vi "Esophogeal_HRME_Main_ImageCasting_VideoCapture.vi"() -> ()   [LabVIEW 2021]
uses:
  typeDefs/Esophogeal_Software_States.ctl
  <vilib>/Utility/miscctls.llb/LVAllMonitorsDisplayTypeDef.ctl
  <vilib>/DAQmx/read.llb/DAQmx Read (Digital 1D Bool NChan 1Samp 1Line).vi
  <extravilib>/ChannelInstances/High Speed Stream-str/_Read For Replicate.vi
  <extravilib>/ChannelInstances/High Speed Stream-a[.,.](u32)/_Read For Replicate.vi
  <extravilib>/ChannelInstances/High Speed Stream-a[.,.](u8)/_Read For Replicate.vi
  <extravilib>/ChannelInstances/Tag-bool/Read With Abort.vi
  <extravilib>/ChannelInstances/Tag-bool/Write With Abort.vi
  <vilib>/DAQmx/create/channels.llb/DAQmx Create Channel (DI-Digital Input).vi
  <vilib>/DAQmx/miscellaneous.llb/DAQmx Fill In Error Info.vi
  <extravilib>/ChannelInstances/Tag-bool/Instantiate.vi
  <extravilib>/ChannelInstances/High Speed Stream-str/Instantiate.vi
  <extravilib>/ChannelInstances/High Speed Stream-a[.,.](u32)/Instantiate.vi
  <extravilib>/ChannelInstances/High Speed Stream-str/)Channel.vi
  <extravilib>/ChannelInstances/High Speed Stream-str/Abort Signal/Init Signal.vi
  <extravilib>/ChannelInstances/High Speed Stream-a[.,.](u32)/)Channel.vi
  <extravilib>/ChannelInstances/High Speed Stream-a[.,.](u32)/Abort Signal/Init Signal.vi
  <extravilib>/ChannelInstances/High Speed Stream-a[.,.](u8)/Instantiate.vi
  <extravilib>/ChannelInstances/High Speed Stream-a[.,.](u8)/)Channel.vi
  <extravilib>/ChannelInstances/High Speed Stream-a[.,.](u8)/Abort Signal/Init Signal.vi
  <extravilib>/ChannelInstances/Tag-bool/EndpointRead.vi
  <extravilib>/ChannelInstances/Tag-bool/Endpoint.vi
  <vilib>/vision/driver/NI_Vision_Acquisition_Software.lvlib
  <resource>/objmgr/imaqdx.rc
  <extravilib>/ChannelInstances/High Speed Stream-a[.,.](u8).lvlib
  <extravilib>/ChannelInstances/High Speed Stream-str.lvlib
  <vilib>/vision/NI_Vision_Development_Module.lvlib
  <extravilib>/ChannelInstances/High Speed Stream-a[.,.](u32).lvlib
  <extravilib>/ChannelInstances/Tag-bool.lvlib
panel:
  out "Pause Status":bool
  in  "Tab Control":enum32{"Main Page", "Image Session Info"}(tab)
  in  "MTN Threshold:":enum16{"15.9", "24.0"}(ring)
  out "Endoscope Feed":T1(plugin-control)
  in  "Calibrate":bool
  out "Image Analysis Meter":dbl(slide) scale=0.0..100.0
  out "Saved Imaged Number":i32=1 caption="Number of Images Saved"
  out "Image Save Notification":string
  in  "Auto Gain":bool=TRUE
  in  "Auto Exposure":bool=TRUE
  in  "Save Button":bool
  out "Recording":bool
  in  "Play Button":bool
  in  "Pause Button":bool
  in  "Close Program":bool
  in  "HRME Gain":dbl(slide)=18.0 scale=0.0..30.0
  in  "HRME Exposure":dbl(slide)=7000.0 scale=100.0..80000.0
  out "HRME Image":T1(plugin-control)
  out "Software States":T2
  out "HRME Path":path
  out "HRME Scores":path
  out "Representative Images":path
  out "error out":errorcluster
  out "Patient Folder":path
  in  "Command File Location":path=path "C:/Users/EsophaHRME_Dell2/Documents/GitHub/Esophageal_HRME_Software/EsophagealDeployment/Multi_Task_Network/CommandFiles/LabVIEW/cmds.json"
  out "Display:All Monitors":T3
  out "Width":i16
  out "Height":i16=960
  out "WideField Path":path
  in  "Python Module Path":path=path "C:/Users/EsophaHRME_Dell2/Documents/GitHub/Esophageal_HRME_Software/EsophagealDeployment/Multi_Task_Network/mainv6.py"
  out "Log File Out":refnum<file>
  out "Timestamp":string
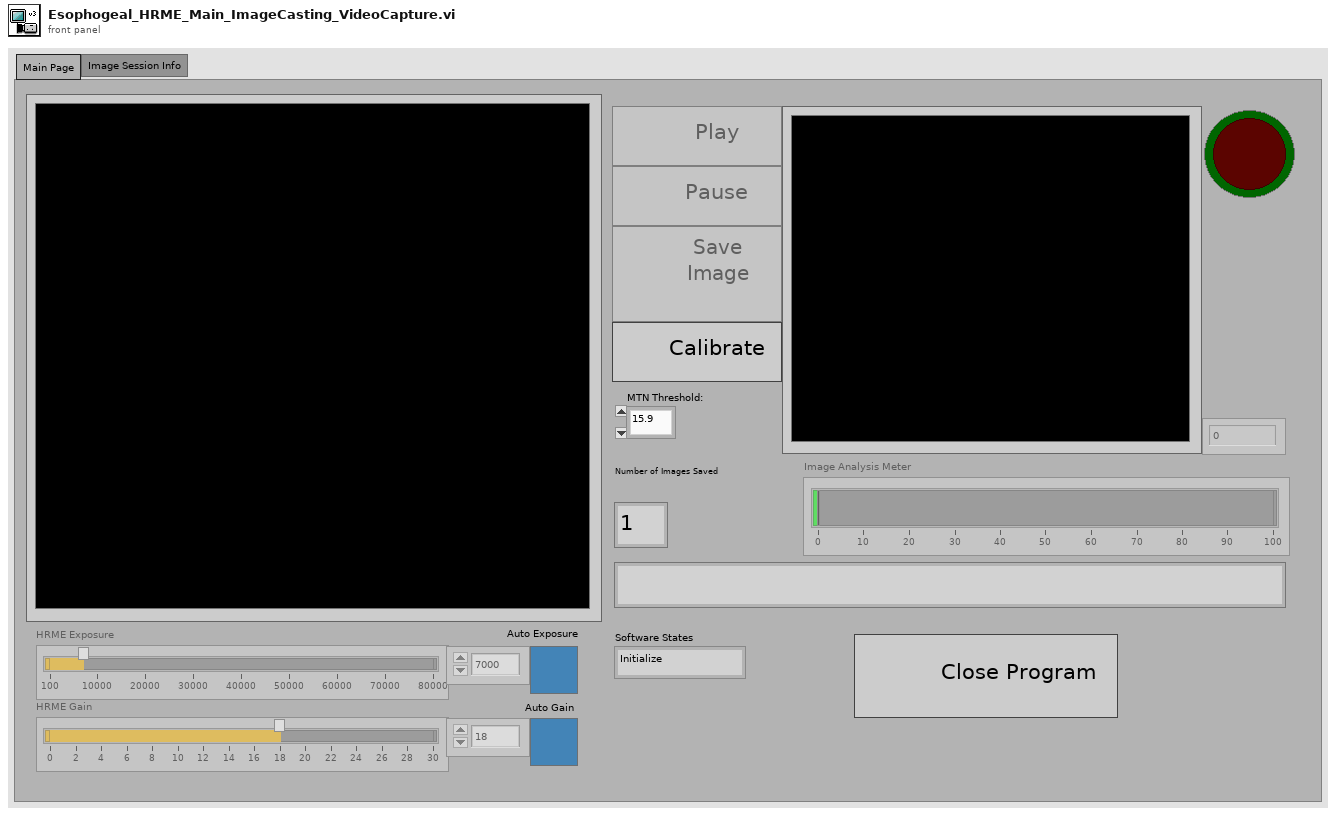
[diagram p1: front panel]
types:
  T1 = typedef "IMAQ Image.ctl" = refnum<image>
  T2 = typedef "Esophogeal_Software_States.ctl" = enum16{"Initialize", "Image Prep Screen", "Imaging", "Image Pause Screen", "Exit"}
  T3 = typedef "LVAllMonitorsDisplayTypeDef.ctl" = cluster{"Bounds":cluster{"Left":i16, "Top":i16, "Right":i16, "Bottom":i16}, "Depth":i16}[]
  T4 = enum8{"Enabled", "Disabled", "Disabled and Grayed Out"}
  T5 = enum16{"open", "replace", "create", "open or create", "replace or create", "replace or create with confirmation"}
  T6 = cluster{"Source":string, "Destination":string, "CMD":string, "Time":string}
  T7 = cluster{"Left":i32, "Top":i32, "Right":i32, "Bottom":i32}
  T8 = typedef "IMAQdx.ctl" = refnum<k21>
  T9 = cluster{"Bounds":cluster{"Left":i16, "Top":i16, "Right":i16, "Bottom":i16}, "Depth":i16}
  T10 = cluster{"Left":i16, "Top":i16, "Right":i16, "Bottom":i16}
  T11 = typedef "Image Type" = u32
  T12 = typedef "ROI Descriptor" = cluster{"Global Rectangle":i32[], "Contours":cluster{"ID":enum32{"External", "Internal"}, "Type":u32, "Coordinates":i32[]}[]}
  T13 = typedef "High Speed Stream-str.lvlib/)Channel.ctl" = refnum<queue>
  T14 = typedef "High Speed Stream-a[.,.](u8).lvlib/)Channel.ctl" = refnum<queue>
  T15 = typedef "Tag-bool.lvlib/))Channel.ctl" = refnum<queue>
  T16 = typedef "High Speed Stream-a[.,.](u32).lvlib/)Channel.ctl" = refnum<queue>
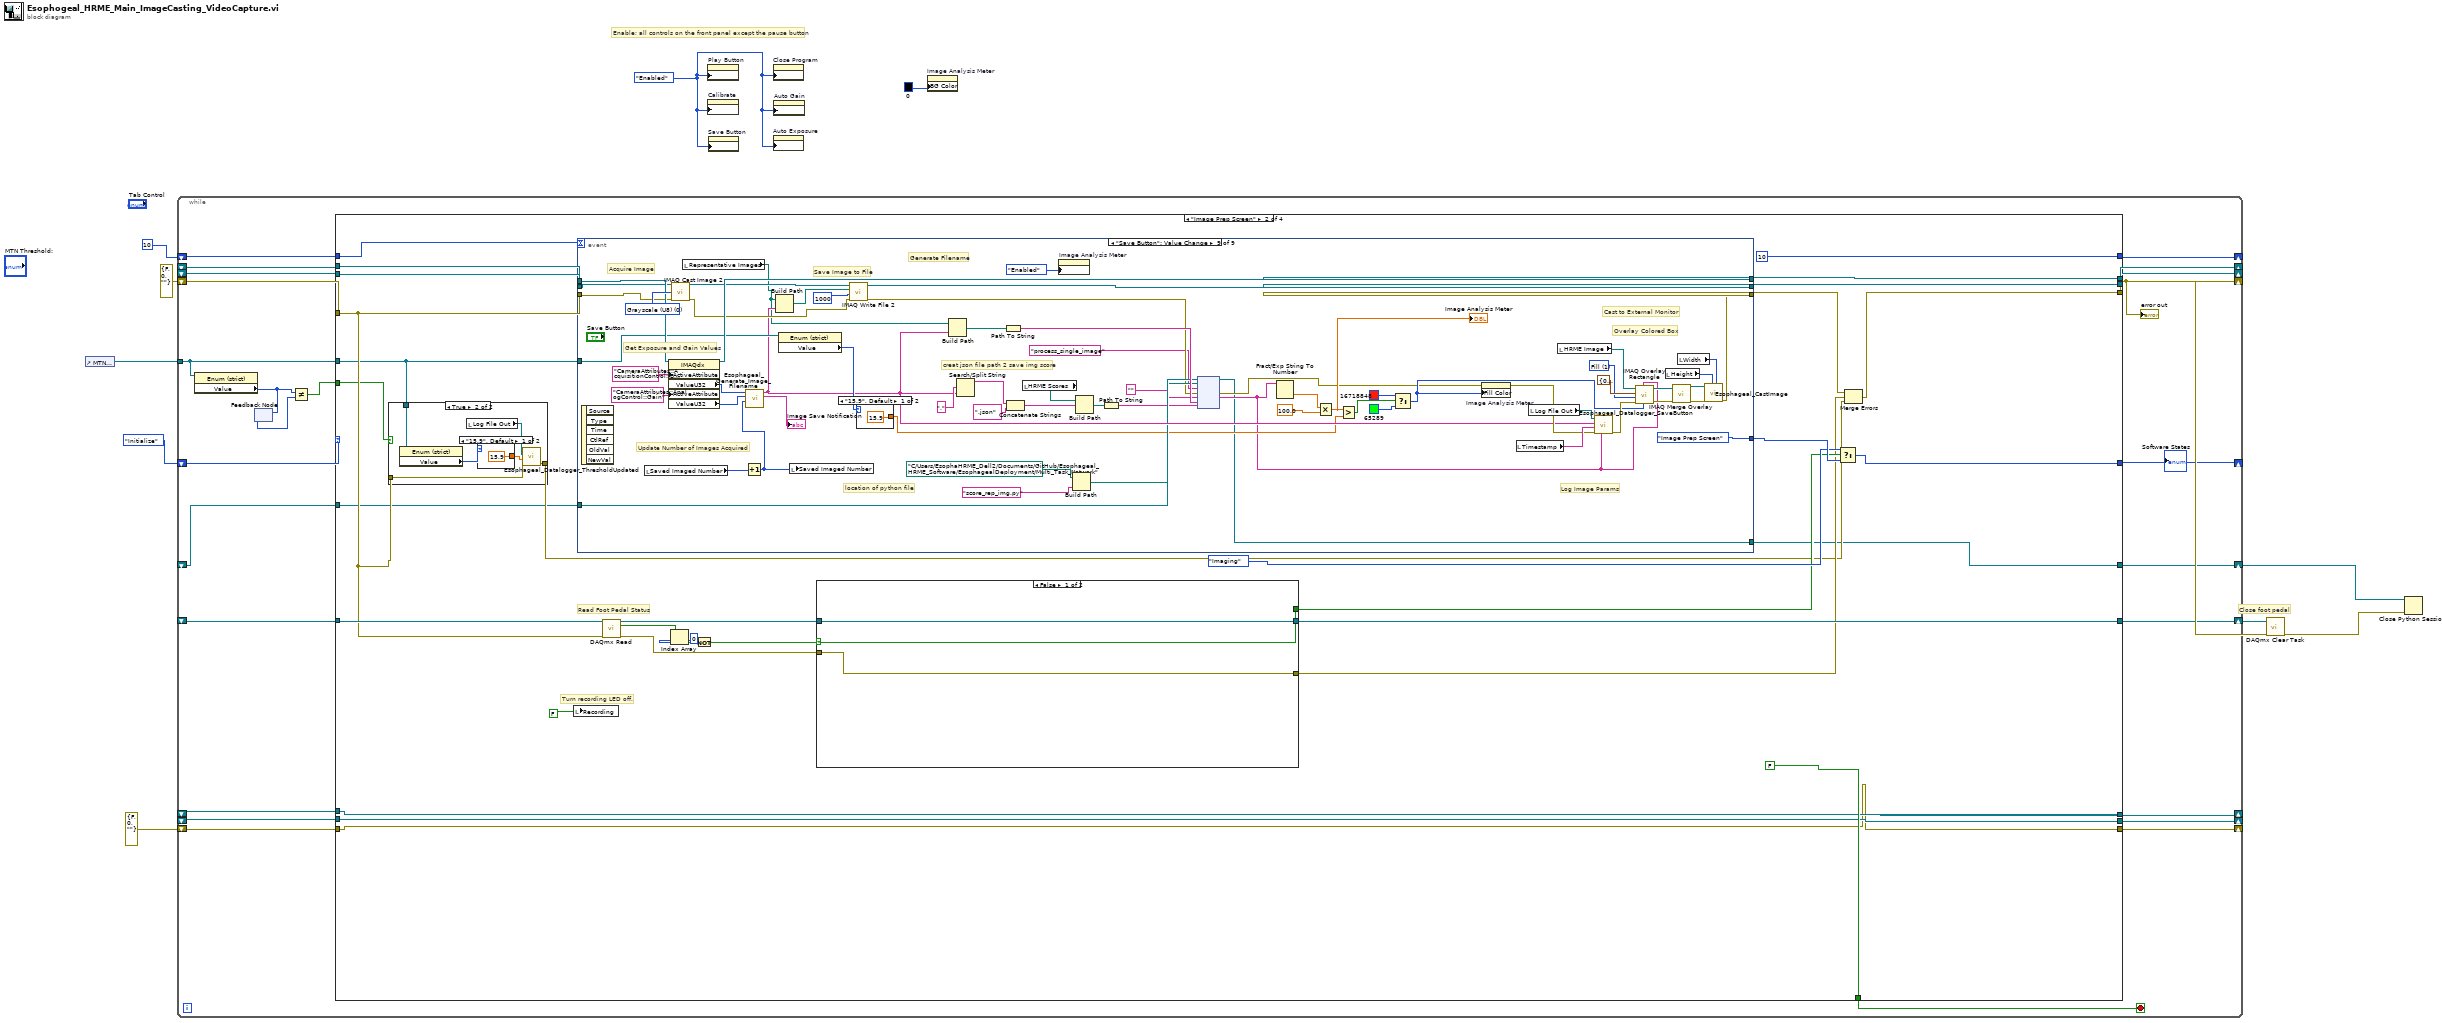
[diagram p0: block diagram]
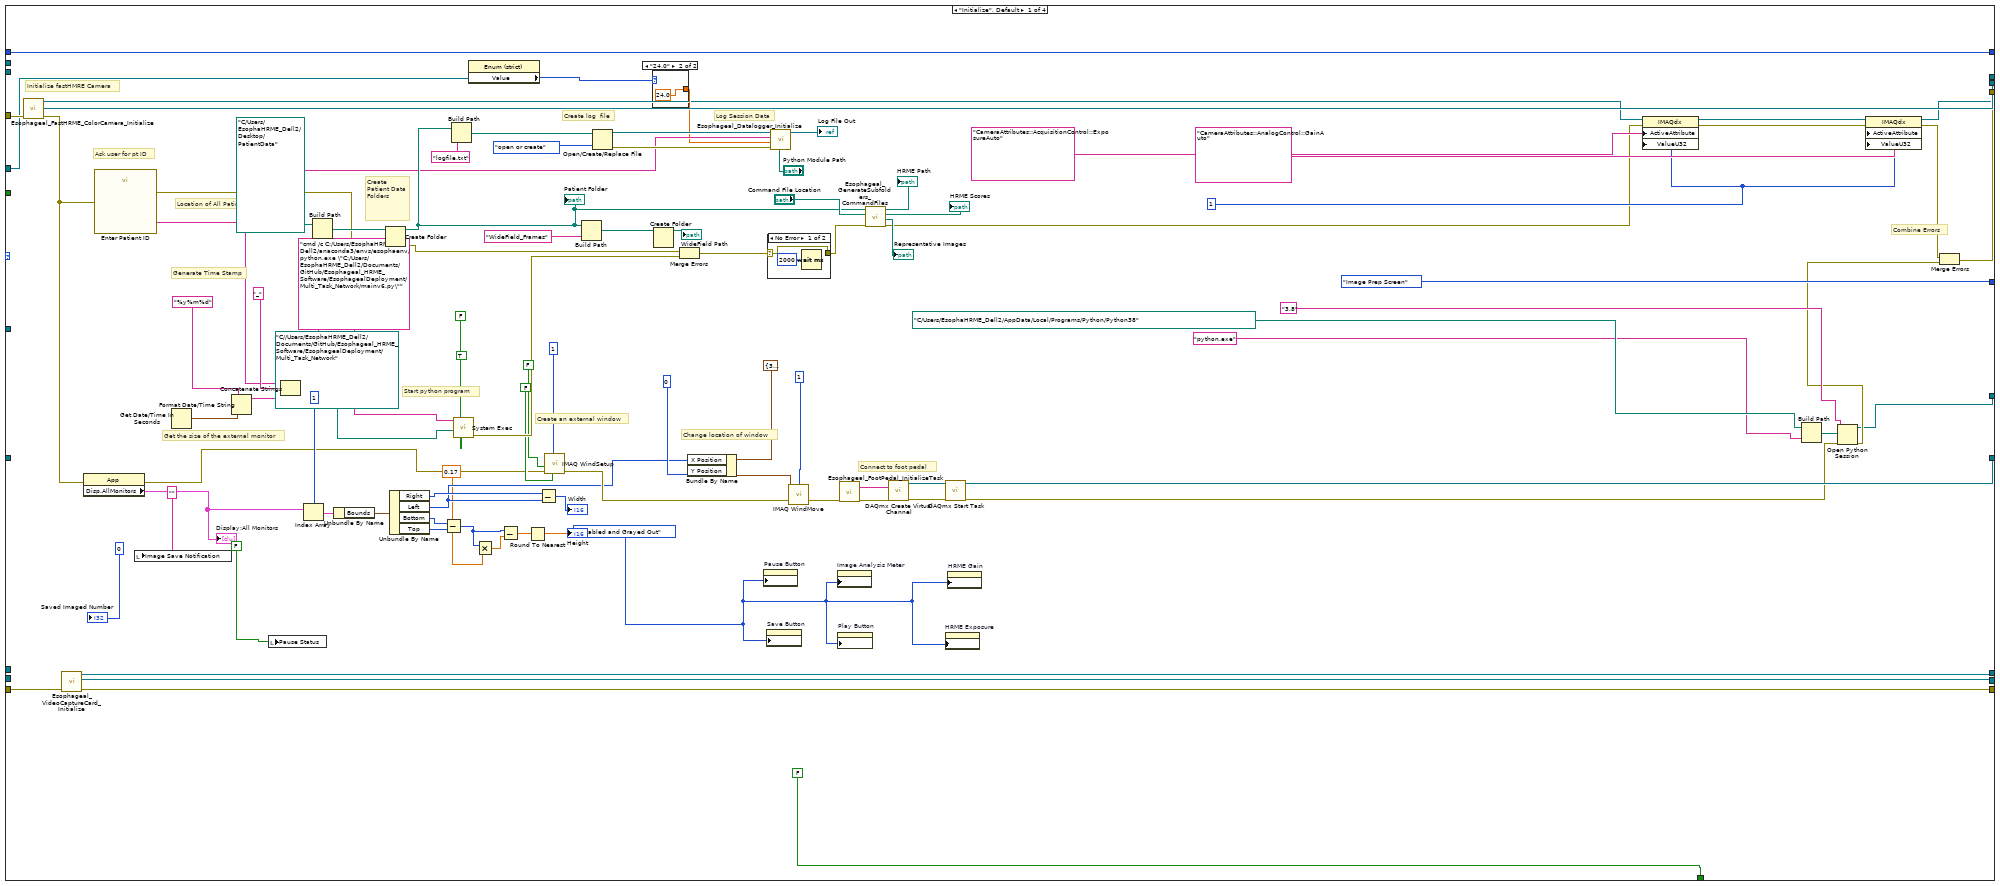
[diagram p2: hidden frame]
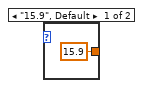
[diagram p3: hidden frame]
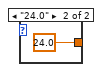
[diagram p6: hidden frame]
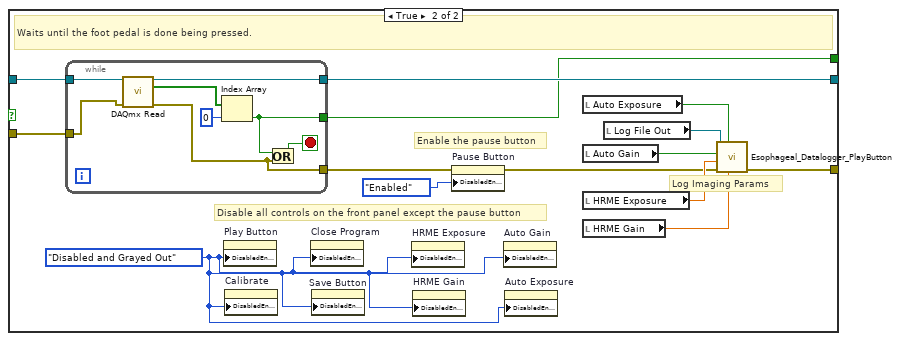
[diagram p7: hidden frame]
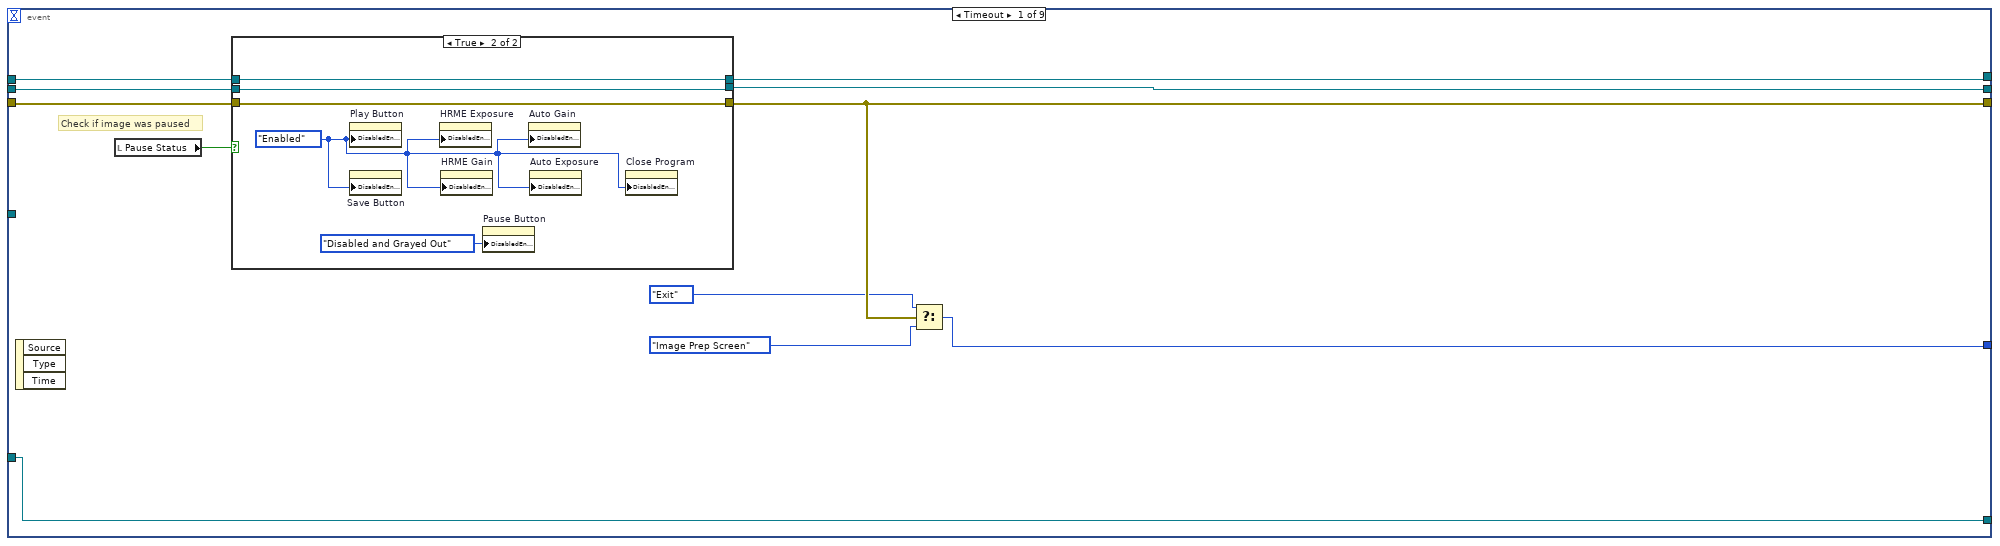
[diagram p8: hidden frame]
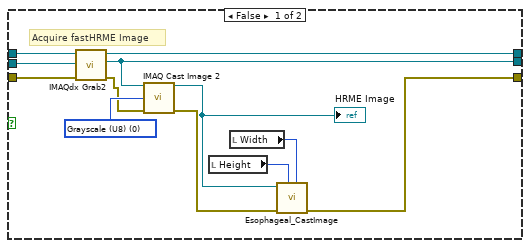
[diagram p9: hidden frame]
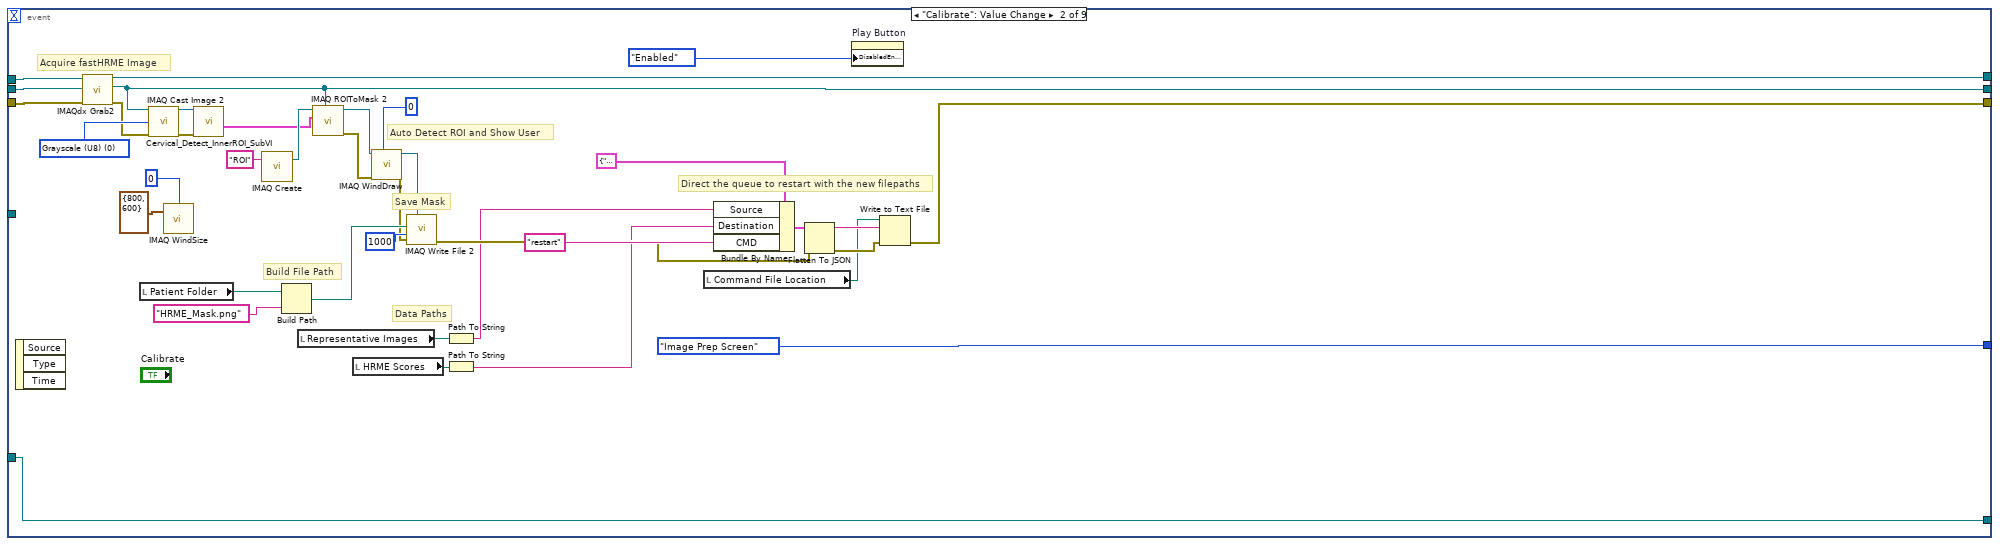
[diagram p10: hidden frame]
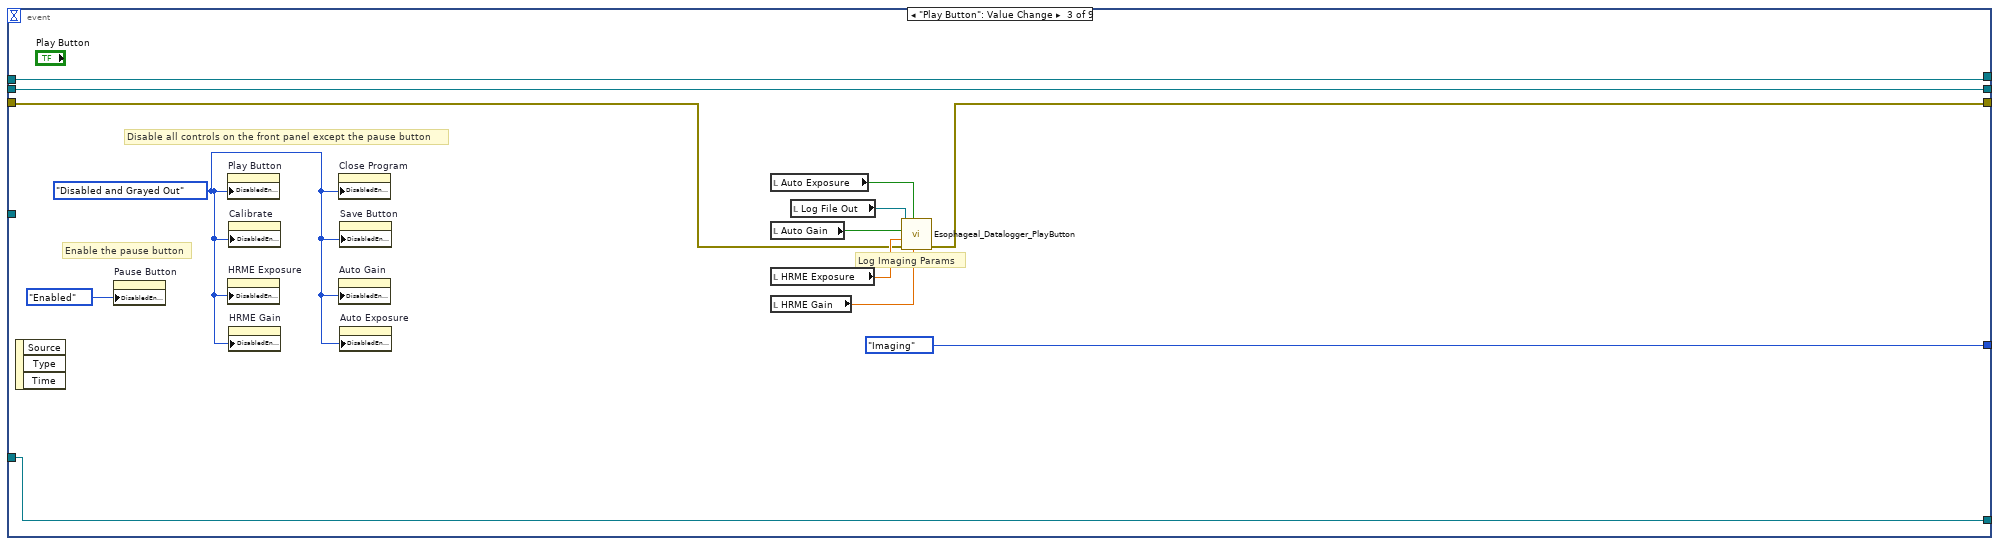
[diagram p11: hidden frame]
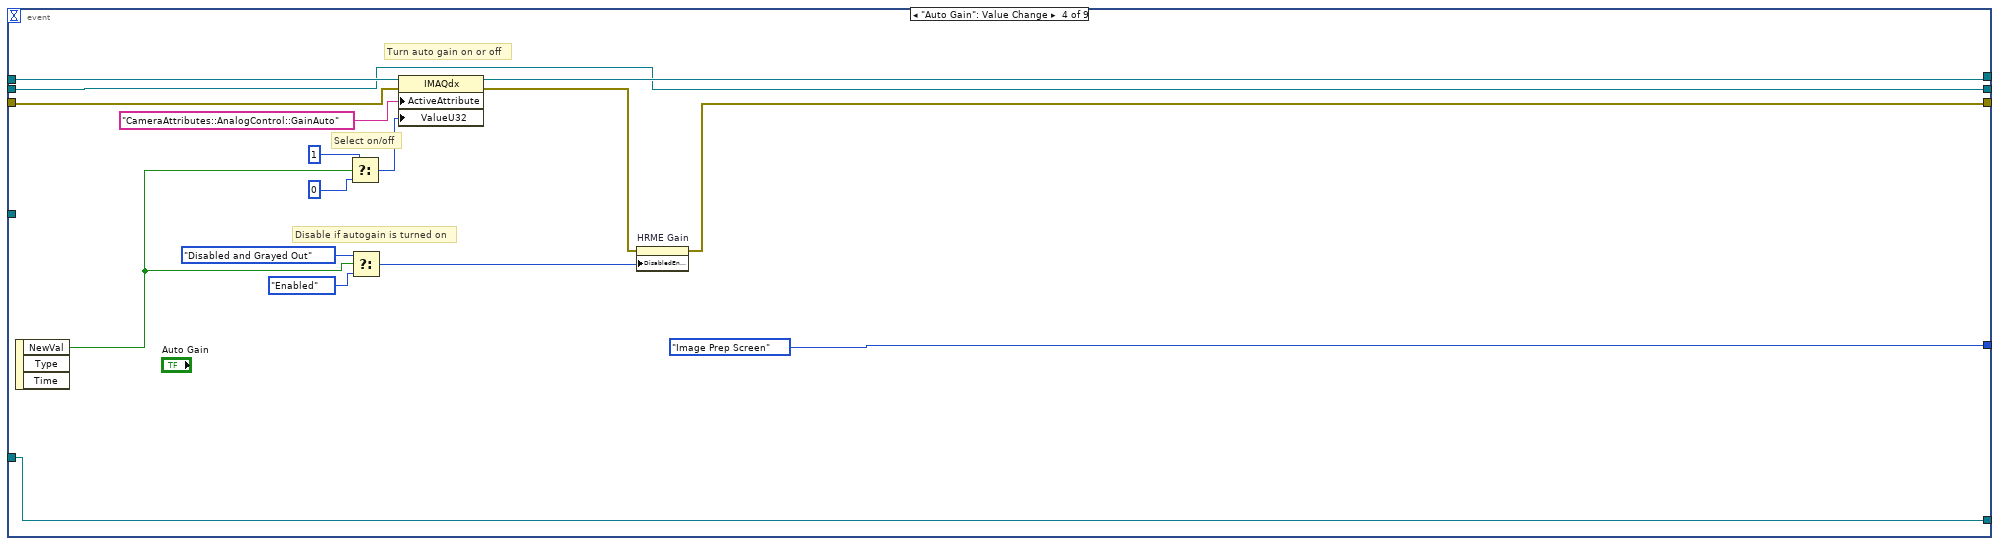
[diagram p12: hidden frame]
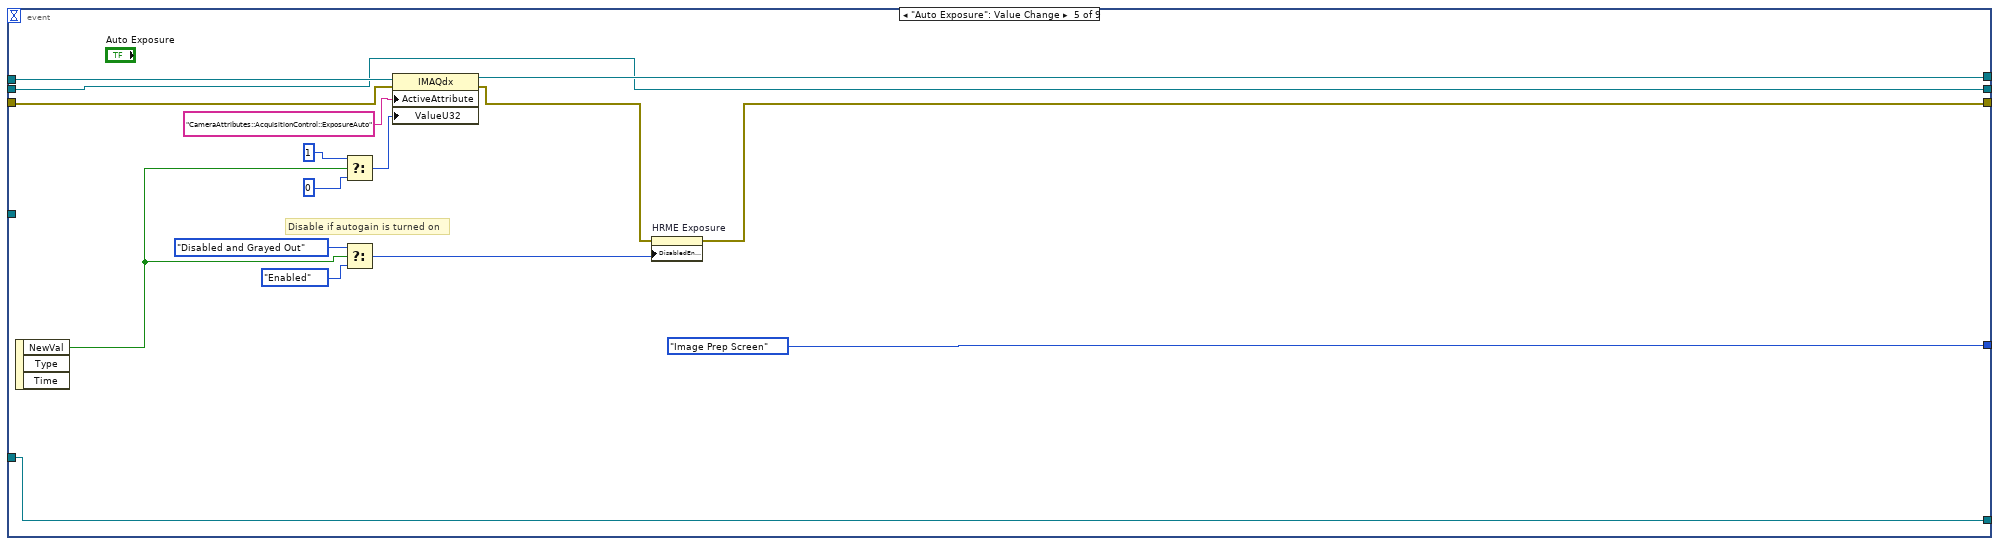
[diagram p13: hidden frame]
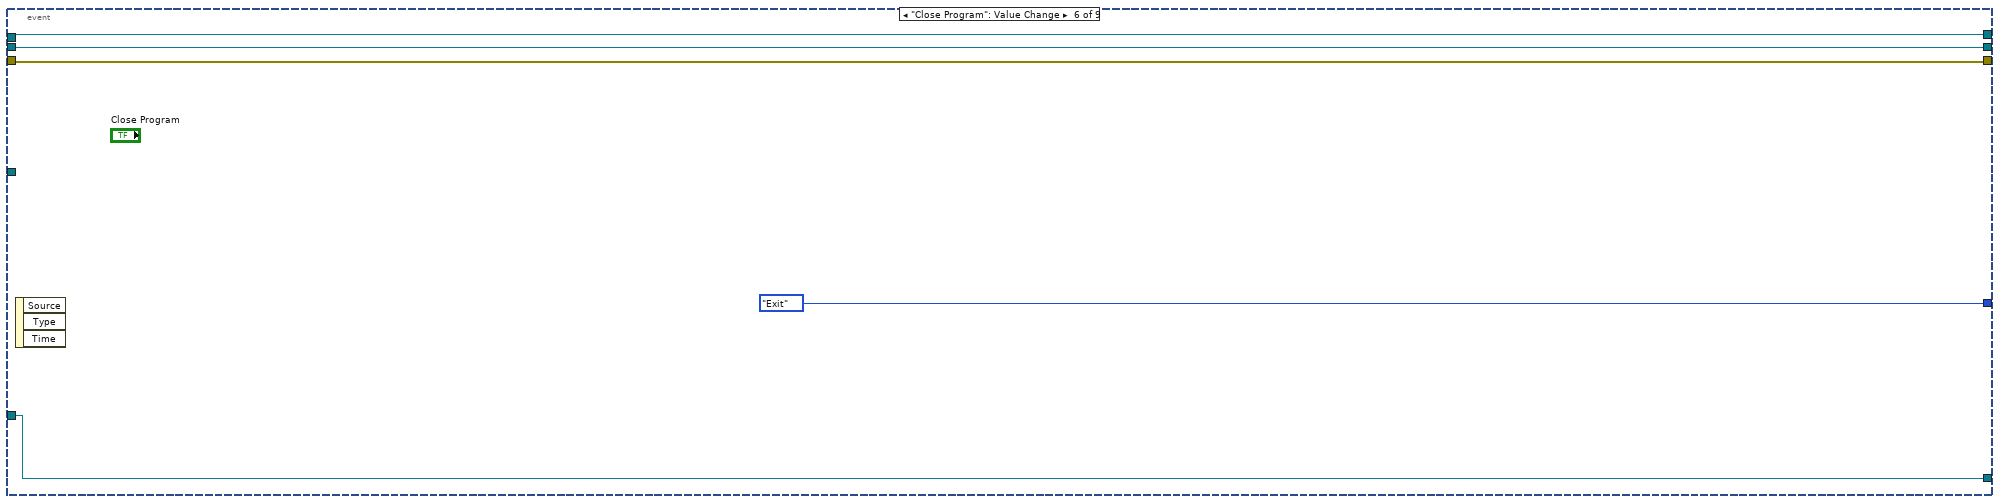
[diagram p14: hidden frame]
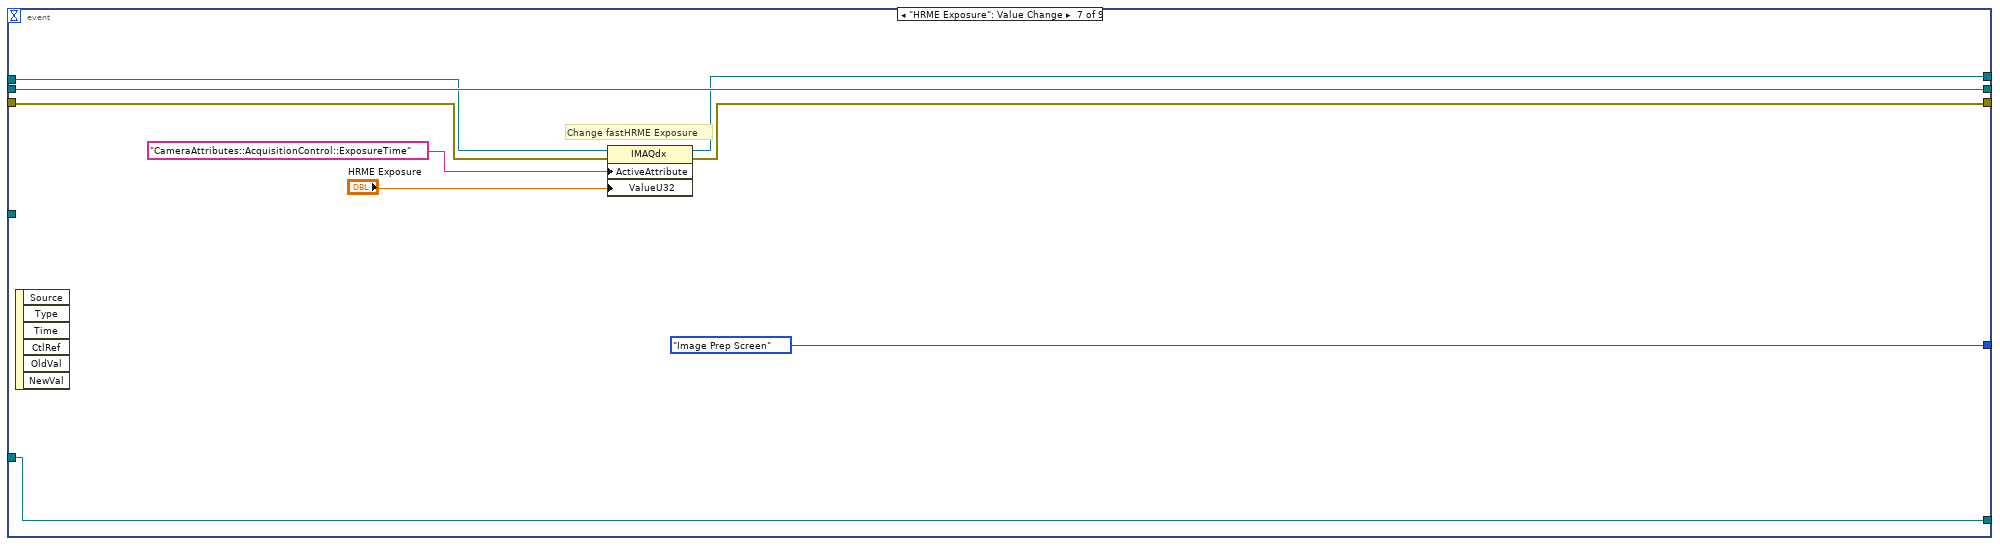
[diagram p15: hidden frame]
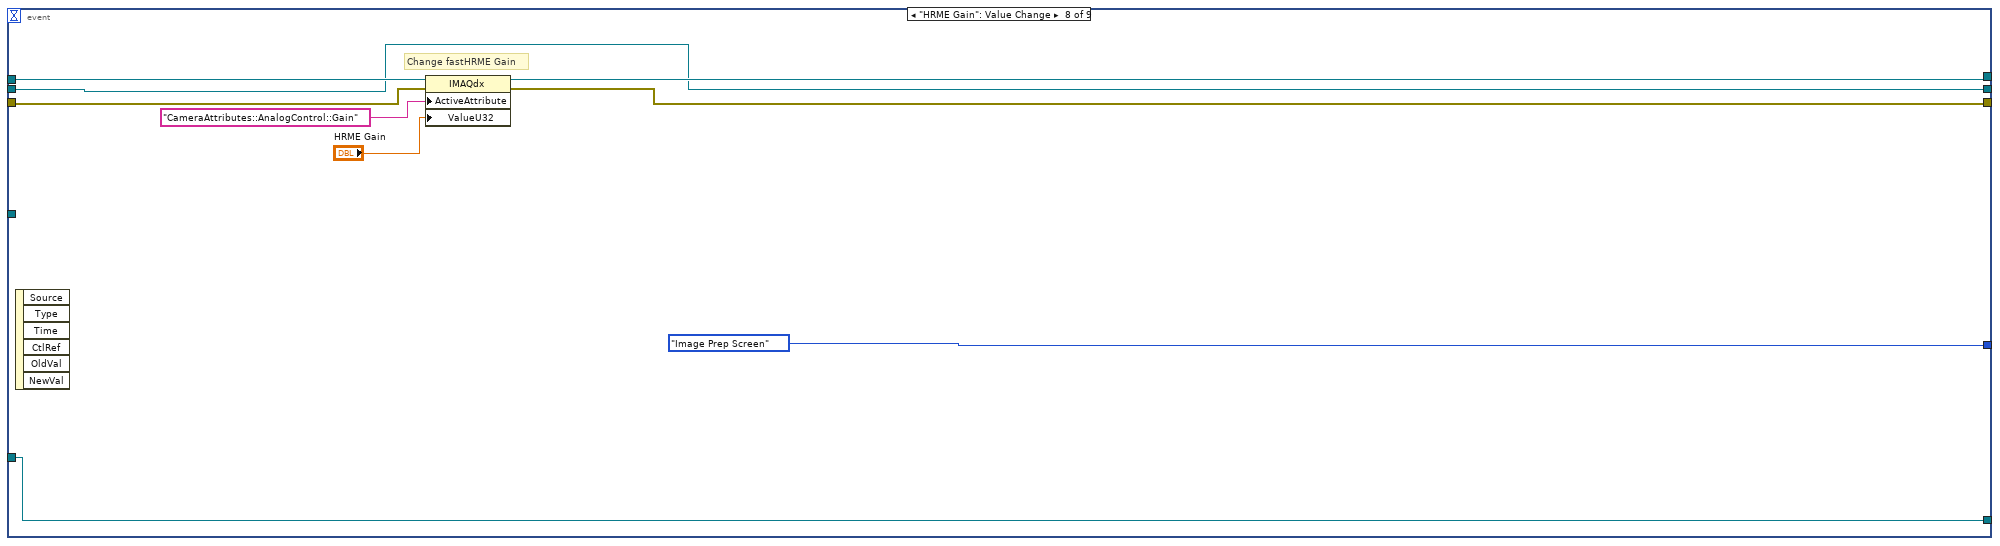
[diagram p16: hidden frame]
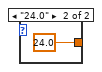
[diagram p17: hidden frame]
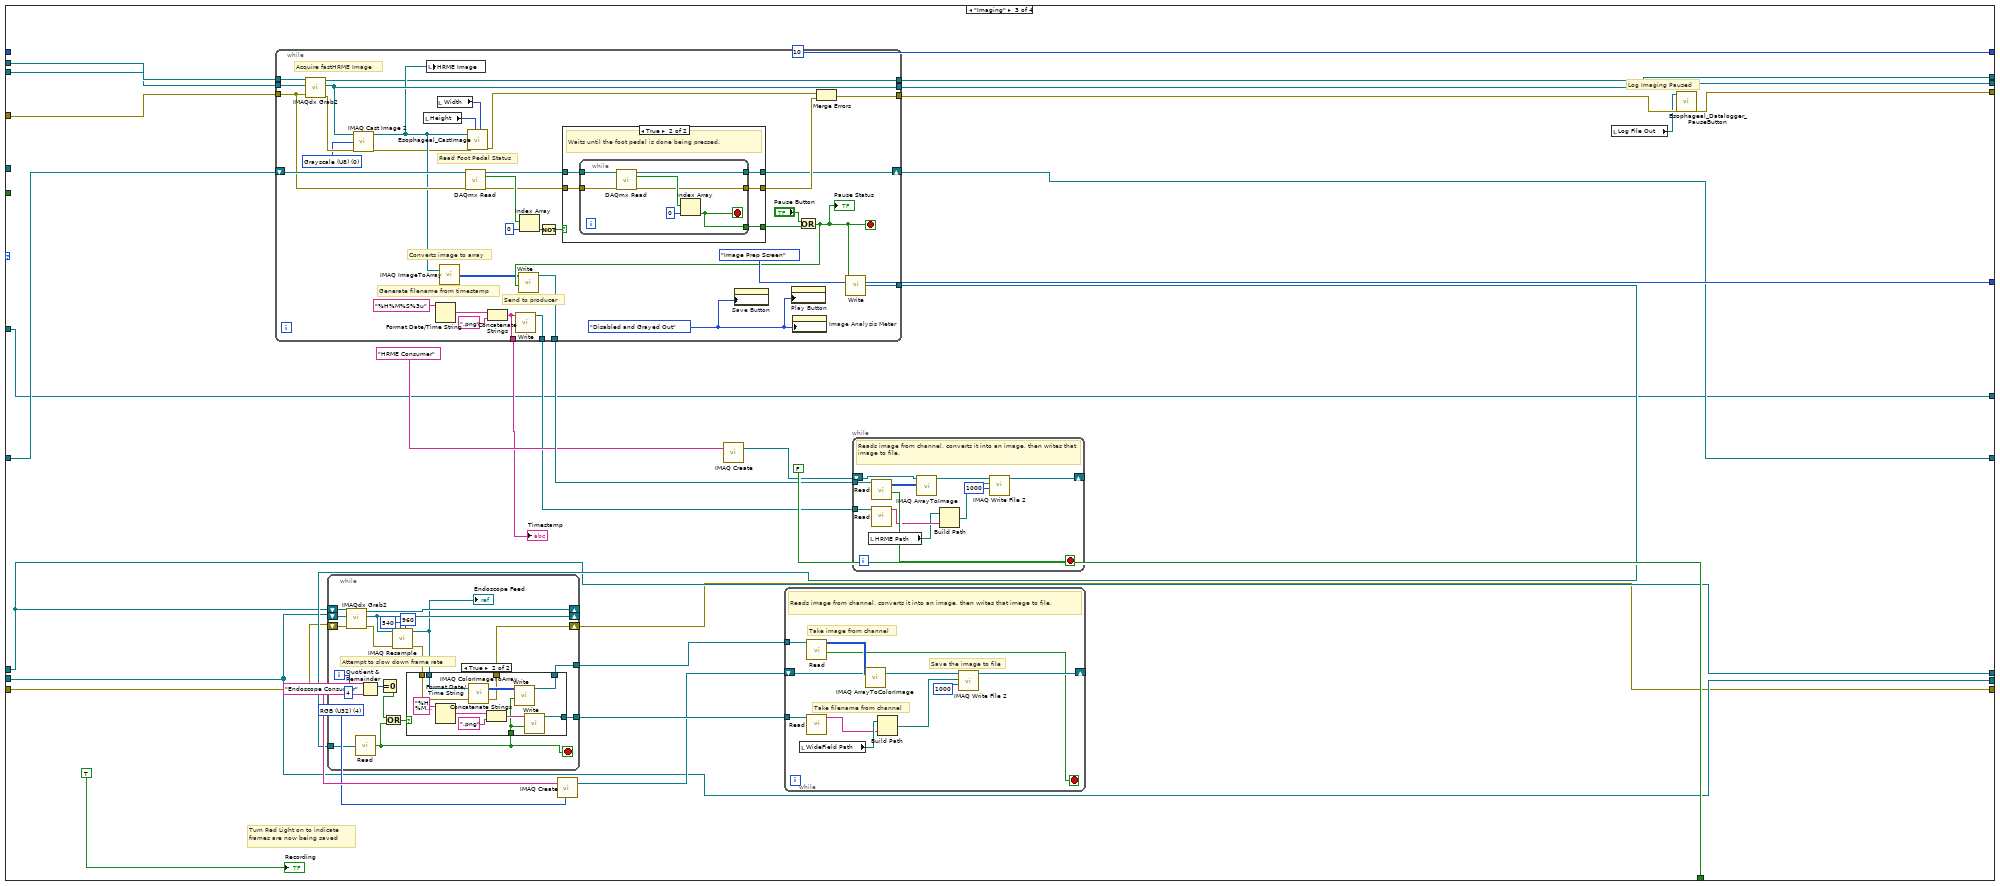
[diagram p18: hidden frame]
diagram:
  w3 = T4."Enabled" ("Disabled")
  # "Enable; all controls on the front panel except the pause button"
  # "Close foot pedal"
  n1 = control-ref of="MTN Threshold:"() -> (w4:refnum<vi>)
  n2 = while {
    shift-right: [w35] -> _
    shift-left: _ -> [w32]
    shift-right: [w34] -> _
    shift-left: _ -> [w31]
    shift-right: [w33] -> _
    shift-left: Esophogeal_Software_States."Initialize" ("Anal HRME States") -> [w36]
    shift-right: [w25] -> w9
    shift-left: errorcluster {"status"=FALSE, "code"=0, "source"=""} ("error IO") -> [w24]
    shift-right: [w28] -> w10
    shift-left: _ -> [w29]
    shift-right: [w26] -> _
    shift-left: 10 -> [w27]
    shift-right: [w21] -> _
    shift-left: _ -> [w22]
    shift-right: [w20] -> _
    shift-left: _ -> [w23]
    shift-right: [w18] -> _
    shift-left: errorcluster {"status"=FALSE, "code"=0, "source"=""} ("error in (no error)") -> [w19]
    tunnel: w4 -> [w17]
    shift-right: [w13] -> w2
    shift-left: _ -> [w12]
    stop <- w30 stop-if-true
    n3 = property class="Enum (strict)"(reference=w17) -> ("Value"=w16:enum16{"15.9", "24.0"})  [unwired: 1 in, 2 out]
    n4 = feedback-in #1(w16) -> ()
    n5 = feedback #1() -> (w15:enum16{"15.9", "24.0"})  [unwired: 1 in]
    n6 = Not Equal?(x=w16, y=w15) -> (x != y?=w14:bool)
    n7 = case shown="\"Image Prep Screen\"" w36 {
      tunnel: [w46 w166 w428 w554] -> w35
      tunnel: [w131 w165 w427 w553] -> w34
      tunnel: [Esophogeal_Software_States."Image Prep Screen" ("Anal HRME States") w162 Esophogeal_Software_States."Image Prep Screen" ("Anal HRME States") Esophogeal_Software_States."Exit" ("Anal HRME States")] -> w33
      tunnel: w24 -> [w129 w142 w412 w543]
      tunnel: w32 -> [_ w168 w430 w554]
      tunnel: w31 -> [_ w167 w429 w553]
      tunnel: [FALSE FALSE FALSE TRUE] -> w30
      tunnel: [w114 w146 w410 w541] -> w25
      tunnel: w29 -> [_ w158 w426 w551]
      tunnel: [w125 w153 w423 w551] -> w28
      tunnel: w27 -> [w124 w151 _ w550]
      tunnel: [w124 10 10 w550] -> w26
      tunnel: w19 -> [w65 w143 w407 w537]
      tunnel: w23 -> [_ w144 w405 w538]
      tunnel: w22 -> [_ w145 w406 w539]
      tunnel: [w62 w144 w405 w538] -> w20
      tunnel: [w63 w145 w406 w539] -> w21
      tunnel: [w64 w143 w404 w537] -> w18
      tunnel: w17 -> [w61 w139 _ _]
      tunnel: w14 -> [_ w140 _ _]
      tunnel: [w37 w137 w403 w536] -> w13
      tunnel: w12 -> [_ w138 w403 w536]
      frame "Initialize", Default {
        w50 = 1
        w44 = T4."Disabled and Grayed Out" ("Disabled")
        # "Log Session Data"
        # "Create log  file"
        # "Change location of window"
        # "Create an external window"
        # "Get the size of the external monitor"
        # "Start python program"
        # "Location of All Patient Data"
        # "Combine Errors"
        # "Create Patient Data Folders"
        # "Generate Time Stamp"
        # "Ask user for pt ID"
        # "Connect to foot pedal"
        # "Initialize fastHMRE Camera"
        n8 = call "Esophageal_FastHRME_ColorCamera_Initialize.vi"("error in (no error)"=w129) -> ("error out"=w91:errorcluster, "HRME Image Reference"=w131:T1, "OMS Camera Reference Out"=w47:T8)  [unwired: 8 in]
        n9 = call "Esophageal_VideoCaptureCard_Initialize.vi"("error in (no error)"=w65) -> ("error out"=w64:errorcluster, "Capture Card Image Out"=w62:T1, "Capture Card Camera Out"=w63:T8)  [unwired: 8 in]
        n10 = property class="App"(error in=w91) -> (error out=w80:errorcluster, "Disp.AllMonitors"=w98:T3)  [unwired: 1 in, 1 out]
        "Display:All Monitors" <- w98
        n11 = call "Enter Patient ID"("error in (no error)"=w91) -> ("Patient ID"=w66:string, "error out"=w115:errorcluster)  [unwired: 16 in, 1 out]
        n12 = local write "Image Save Notification"("" ("Image Save Notification")) -> ()
        n13 = Get Date/Time In Seconds() -> (seconds since 1Jan1904=w121:timestamp)
        n14 = Format Date/Time String(time format string (%c)="%y%m%d", seconds (now)=w121) -> (date/time string=w118:string)  [unwired: 1 in]
        n15 = local write "Pause Status"(FALSE ("Pause Status")) -> ()
        n16 = Concatenate Strings(w66, "_" ("string"), w118) -> (w117:string)
        n17 = Index Array(array=w98, index=1) -> (element=w96:T9)
        n18 = Build Path(base path=path "C:/Users/EsophaHRME_Dell2/Desktop/PatientData", name or relative path=w117) -> (appended path=w116:path)
        n19 = Unbundle By Name(w96) -> ("Bounds"=w95:T10)
        n20 = Create Folder(path (use dialog)=w116, error in=w115) -> (created path=w68:path, error out=w78:errorcluster)  [unwired: 1 in, 1 out]
        "Patient Folder" <- w68
        n21 = Unbundle By Name(w95) -> ("Right"=w94:i16, "Left"=w79:i16, "Bottom"=w93:i16, "Top"=w92:i16)
        n22 = Subtract(x=w93, y=w92) -> (x-y=w57:i16)
        n23 = Build Path(base path=w68, name or relative path="logfile.txt") -> (appended path=w74:path)
        n24 = call <vilib>:"System Exec.vi"("run minimized? (F)"=TRUE, "wait until completion? (T)"=FALSE, "working directory"=path "C://Users/EsophaHRME_Dell2/Documents/GitHub/Esophageal_HRME_Software/EsophagealDeployment/Multi_Task_Network", "command line"="cmd /c C:/Users/EsophaHRME_Dell2/anaconda3/envs/esophaenv/python.exe \"C:/Users/EsophaHRME_Dell2/Documents/GitHub/Esophageal_HRME_Software/EsophagealDeployment/Multi_Task_Network/mainv6.py\"") -> ("error out"=w103:errorcluster)  [unwired: 4 in, 3 out]
        n25 = property class="Enum (strict)"(reference=w61) -> ("Value"=w60:enum16{"15.9", "24.0"})  [unwired: 1 in, 2 out]
        n26 = Multiply(x=w57, y=0.17) -> (x*y=w56:dbl)
        n27 = Subtract(x=w57, y=w56) -> (x-y=w55:dbl)
        n28 = Round To Nearest(number=w55) -> (nearest integer value=→"Height":dbl)
        n29 = Subtract(x=w94, y=w79) -> (x-y=→"Width":i16)
        n30 = call "IMAQ WindSetup"("Window is floating? (No)"=FALSE, "Window Number (0...15)"=1, "error in (no error)"=w80, "Window has title bar? (Yes)"=FALSE) -> ("error out"=w81:errorcluster)  [unwired: 7 in]
        n31 = Build Path(base path=w68, name or relative path="WideField_Frames") -> (appended path=w76:path)
        n32 = Open/Create/Replace File(file path (use dialog)=w74, operation (0:open)=T5."open or create") -> (refnum out=w72:refnum<file>, error out=w71:errorcluster)  [unwired: 4 in, 1 out]
        n33 = case shown="\"24.0\"" w60 {
          tunnel: [15.9 24.0] -> w59
          frame "15.9", Default {
          }
          frame "24.0" {
          }
        }
        n34 = Create Folder(path (use dialog)=w76) -> (created path=→"WideField Path":path)  [unwired: 2 in, 2 out]
        n35 = Merge Errors(w78, w103) -> (w104:errorcluster)
        n36 = Bundle By Name(cluster=cluster{"X Position":i32, "Y Position":i32} {"X Position"=3840, "Y Position"=0} ("Coordinates (screen)"), "X Position"=w79, "Y Position"=0) -> (w86:cluster{"X Position":i32, "Y Position":i32})
        n37 = property on="Pause Button" class="Bool"("DisabledEnum"=w44) -> ()  [unwired: 2 in, 2 out]
        n38 = property on="Save Button" class="Bool"("DisabledEnum"=w44) -> ()  [unwired: 2 in, 2 out]
        n39 = case shown="No Error" w104 {
          selector: w104 -> [w134 w136]
          tunnel: [w134 w136] -> w108
          frame No Error {
            n40 = Wait (ms)(milliseconds to wait=u32 2000) -> ()  [unwired: 1 out]
          }
          frame Error {
          }
        }
        n41 = call "Esophageal_Datalogger_Initialize.vi"("Python Module Path"="Python Module Path", "error in (no error)"=w71, "MTN Threshold"=w59, "Patient ID"=w66, "Log File In"=w72) -> ("Log File Out"=→"Log File Out":refnum<file>)  [unwired: 5 in, 1 out]
        n42 = call "IMAQ WindMove"("Window Number (0...15)"=1, "Coordinates (screen)"=w86, "error in (no error)"=w81) -> ("error out"=w82:errorcluster)  [unwired: 2 in, 1 out]
        n43 = property on="Image Analysis Meter" class="Slide (strict)"("DisabledEnum"=w44) -> ()  [unwired: 2 in, 2 out]
        n44 = property on="Play Button" class="Bool"("DisabledEnum"=w44) -> ()  [unwired: 2 in, 2 out]
        n45 = call "Esophageal_FootPedal_InitializeTask.vi"("error in (no error)"=w82) -> ("error out"=w101:errorcluster, "Task Command"=w100:string)  [unwired: 9 in]
        n46 = call "Esophageal_GenerateSubfolders_CommandFiles.vi"("error in"=w108, "Command File Location"="Command File Location", "Patient Data Folder"=w68) -> ("error out"=w48:errorcluster, "Rep Image Path"=→"Representative Images":path, "HRME Scores"=→"HRME Scores":path, "HRME Path"=→"HRME Path":path)  [unwired: 5 in]
        n47 = call-poly <vilib>:"DAQmx Create Virtual Channel.vi"("lines"=w100, "error in"=w101) -> ("task out"=w126:refnum<k21>, "error out"=w127:errorcluster)  [unwired: 12 in]
        n48 = property on="HRME Exposure" class="Slide (strict)"("DisabledEnum"=w44) -> ()  [unwired: 2 in, 2 out]
        n49 = call <vilib>:"DAQmx Start Task.vi"("task/channels in"=w126, "error in"=w127) -> ("task out"=w125:refnum<k21>, "error out"=w39:errorcluster)  [unwired: 12 in]
        n50 = property on="HRME Gain" class="Slide (strict)"("DisabledEnum"=w44) -> ()  [unwired: 2 in, 2 out]
        n51 = property class="IMAQdx"(reference=w47, error in=w48, "ActiveAttribute"="CameraAttributes::AcquisitionControl::ExposureAuto", "ValueU32"=w50) -> (reference out=w49:T8, error out=w51:errorcluster)
        n52 = Build Path(base path=path "C:/Users/EsophaHRME_Dell2/AppData/Local/Programs/Python/Python38", name or relative path="python.exe") -> (appended path=w42:path)
        n53 = Open Python Session(python version="3.8", python path=w42, 3:w39) -> (session out=w37:refnum<k35>, error out=w38:errorcluster)
        n54 = property class="IMAQdx"(reference=w49, error in=w51, "ActiveAttribute"="CameraAttributes::AnalogControl::GainAuto", "ValueU32"=w50) -> (reference out=w46:T8, error out=w45:errorcluster)
        n55 = Merge Errors(w45, w38) -> (w114:errorcluster)
        "Saved Imaged Number" <- 0
      }
      frame "Image Prep Screen" {
        # "Turn recording LED off."
        # "Read Foot Pedal Status"
        n56 = case shown="True" w140 {
          tunnel: w142 -> [w169 w173]
          tunnel: [w169 w172] -> w141
          tunnel: w139 -> [_ w170]
          frame False {
          }
          frame True {
            n57 = property class="Enum (strict)"(reference=w170) -> ("Value"=w175:enum16{"15.9", "24.0"})  [unwired: 1 in, 2 out]
            n58 = local read "Log File Out"() -> (w171:refnum<file>)
            n59 = case shown="\"15.9\", Default" w175 {
              tunnel: [15.9 24.0] -> w174
              frame "15.9", Default {
              }
              frame "24.0" {
              }
            }
            n60 = call "Esophageal_Datalogger_ThresholdUpdated.vi"("error in"=w173, "MTN Threshold"=w174, "Log File In"=w171) -> ("error out"=w172:errorcluster)  [unwired: 7 in, 1 out]
          }
        }
        n61 = local write "Recording"(FALSE ("Recording")) -> ()
        n62 = event shown="[8] \"Save Button\": Value Change" {
          selector: _ -> [_ _ _ _ _ _ _ _ _]
          dyn-events: _ -> [_ _ _ _ _ _ _ _ _]
          timeout: w151 -> [_ _ _ _ _ _ _ _ _]
          tunnel: w168 -> [w213 w267 w280 w297 w310 w317 w325 w334 w385]
          tunnel: w167 -> [w211 w266 w279 w294 w307 w316 w326 w330 w384]
          tunnel: [w205 Esophogeal_Software_States."Image Prep Screen" ("Anal HRME States") Esophogeal_Software_States."Imaging" ("Anal HRME States") Esophogeal_Software_States."Image Prep Screen" ("Anal HRME States") Esophogeal_Software_States."Image Prep Screen" ("Anal HRME States") Esophogeal_Software_States."Exit" ("Anal HRME States") Esophogeal_Software_States."Image Prep Screen" ("Anal HRME States") Esophogeal_Software_States."Image Prep Screen" ("Anal HRME States") Esophogeal_Software_States."Image Prep Screen" ("Anal HRME States")] -> w161
          tunnel: [w212 w264 w280 w296 w309 w317 w324 w333 w395] -> w166
          tunnel: [w210 w242 w279 w294 w307 w316 w326 w330 w398] -> w165
          tunnel: w142 -> [w209 w265 w271 w295 w308 w315 w321 w331 w383]
          tunnel: [w206 w250 w270 w285 w303 w315 w320 w332 w380] -> w147
          tunnel: w139 -> [_ _ _ _ _ _ _ _ w367]
          tunnel: w138 -> [w203 w231 w269 w282 w298 w314 w319 w328 w353]
          tunnel: [w203 w231 w269 w282 w298 w314 w319 w328 w337] -> w137
          event Timeout {
            # "Check if image was paused"
            n63 = event-data() -> ()  [unwired: 1 in, 3 out]
            n64 = local read "Pause Status"() -> (w208:bool)
            n65 = case shown="True" w208 {
              tunnel: w213 -> [w225 w230]
              tunnel: [w224 w230] -> w212
              tunnel: w211 -> [w223 w229]
              tunnel: [w221 w229] -> w210
              tunnel: w209 -> [w222 w227]
              tunnel: [w216 w227] -> w206
              frame False {
                w220 = T11 0 items=["Grayscale (U8)", "Grayscale (I16)", "Grayscale (SGL)", "Complex (CSG)", "RGB (U32)", "HSL (U32)", "RGB (U64)", "Grayscale (U16)"] ("Image Type")
                # "Acquire fastHRME Image"
                n66 = call <vilib>:"IMAQdx Grab2.vi"("error in"=w222, "Image In"=w223, "Session In"=w225) -> ("error out"=w218:errorcluster, "Image Out"=w221:T1, "Session Out"=w224:T8)  [unwired: 5 in, 1 out]
                n67 = call "IMAQ Cast Image 2"("Image Src"=w221, "Image Type"=w220, "error in (no error)"=w218) -> ("Image Dst Out"=w219:T1, "error out"=w217:errorcluster)  [unwired: 11 in]
                "HRME Image" <- w219
                n68 = local read "Height"() -> (w215:i16)
                n69 = local read "Width"() -> (w214:i16)
                n70 = call "Esophageal_CastImage.vi"("X Resolution"=w214, "Y Resolution"=w215, "error in (no error)"=w217, "Image In"=w219) -> ("error out"=w216:errorcluster)  [unwired: 7 in]
              }
              frame True {
                w226 = T4."Enabled" ("Disabled")
                n71 = property on="Play Button" class="Bool"("DisabledEnum"=w226) -> ()  [unwired: 2 in, 2 out]
                n72 = property on="Save Button" class="Bool"("DisabledEnum"=w226) -> ()  [unwired: 2 in, 2 out]
                n73 = property on="HRME Exposure" class="Slide (strict)"("DisabledEnum"=w226) -> ()  [unwired: 2 in, 2 out]
                n74 = property on="HRME Gain" class="Slide (strict)"("DisabledEnum"=w226) -> ()  [unwired: 2 in, 2 out]
                n75 = property on="Pause Button" class="Bool"("DisabledEnum"=T4."Disabled and Grayed Out" ("Disabled")) -> ()  [unwired: 2 in, 2 out]
                n76 = property on="Auto Gain" class="Bool (strict)"("DisabledEnum"=w226) -> ()  [unwired: 2 in, 2 out]
                n77 = property on="Auto Exposure" class="Bool (strict)"("DisabledEnum"=w226) -> ()  [unwired: 2 in, 2 out]
                n78 = property on="Close Program" class="Bool"("DisabledEnum"=w226) -> ()  [unwired: 2 in, 2 out]
              }
            }
            n79 = Select(t=Esophogeal_Software_States."Exit" ("Anal HRME States"), s=w206, f=Esophogeal_Software_States."Image Prep Screen" ("Anal HRME States")) -> (s? t:f=w205:T2)
          }
          event "Calibrate": Value Change {
            w268 = T11 0 items=["Grayscale (U8)", "Grayscale (I16)", "Grayscale (SGL)", "Complex (CSG)", "RGB (U32)", "HSL (U32)", "RGB (U64)", "Grayscale (U16)"] ("Image Type")
            # "Auto Detect ROI and Show User"
            # "Data Paths"
            # "Direct the queue to restart with the new filepaths"
            # "Build File Path"
            # "Save Mask"
            # "Acquire fastHRME Image"
            n80 = event-data() -> ()  [unwired: 1 in, 3 out]
            n81 = call <vilib>:"IMAQdx Grab2.vi"("error in"=w265, "Image In"=w266, "Session In"=w267) -> ("error out"=w256:errorcluster, "Image Out"=w242:T1, "Session Out"=w264:T8)  [unwired: 5 in, 1 out]
            n82 = local read "Patient Folder"() -> (w262:path)
            n83 = call "IMAQ Cast Image 2"("Image Src"=w242, "Image Type"=w268, "error in (no error)"=w256) -> ("Image Dst Out"=w233:T1, "error out"=w234:errorcluster)  [unwired: 11 in]
            n84 = call "IMAQ WindSize"("Width & Height"=cluster{"Width":i32, "Height":i32} {"Width"=800, "Height"=600}, "Window Number"=0) -> ()  [unwired: 4 in, 3 out]
            n85 = call "Cervical_Detect_InnerROI_SubVI.vi"("error in"=w234, "Raw Image"=w233) -> ("ROI Descriptor"=w232:T12)  [unwired: 6 in, 3 out]
            n86 = call "IMAQ Create"("Image Name"="ROI") -> ("New Image"=w257:T1)  [unwired: 4 in, 1 out]
            n87 = Build Path(base path=w262, name or relative path="HRME_Mask.png") -> (appended path=w260:path)
            n88 = local read "Representative Images"() -> (w247:path)
            n89 = call "IMAQ ROIToMask 2"("Image Model"=w242, "ROI Descriptor"=w232, "Image"=w257) -> ("error out"=w237:errorcluster, "Image Out"=w238:T1)  [unwired: 6 in, 1 out]
            n90 = local read "HRME Scores"() -> (w246:path)
            n91 = call "IMAQ WindDraw"("Window Number (0...15)"=0, "error in (no error)"=w237, "Image"=w238) -> ("error out"=w235:errorcluster, "Image Out (duplicate)"=w236:T1)  [unwired: 7 in]
            n92 = call-poly "IMAQ Write File 2"("error in (no error)"=w235, "Image Quality"=u32 1000, "File Path"=w260, "Image"=w236) -> ("error out"=w252:errorcluster)  [unwired: 6 in, 1 out]
            n93 = Path To String(path=w247) -> (string=w245:string)
            n94 = Path To String(path=w246) -> (string=w244:string)
            n95 = local read "Command File Location"() -> (w248:path)
            n96 = Bundle By Name(cluster=T6 {"Source"="", "Destination"="", "CMD"="newfolders", "Time"="time"} ("Output JSON File"), "Source"=w245, "Destination"=w244, "CMD"="restart") -> (w254:T6)
            n97 = Flatten To JSON(anything=w254, error in (no error)=w252) -> (JSON string=w255:string, 11:w251:errorcluster)  [unwired: 1 in]
            n98 = property on="Play Button" class="Bool"("DisabledEnum"=T4."Enabled" ("Disabled")) -> ()  [unwired: 2 in, 2 out]
            n99 = Write to Text File(file (use dialog)=w248, text=w255, error in=w251) -> (error out=w250:errorcluster)  [unwired: 1 in, 2 out]
          }
          event "Play Button": Value Change {
            w277 = T4."Disabled and Grayed Out" ("Disabled")
            # "Log Imaging Params"
            # "Enable the pause button"
            # "Disable all controls on the front panel except the pause button"
            n100 = event-data() -> ()  [unwired: 1 in, 3 out]
            n101 = property on="Pause Button" class="Bool"("DisabledEnum"=T4."Enabled" ("Disabled")) -> ()  [unwired: 2 in, 2 out]
            n102 = property on="Play Button" class="Bool"("DisabledEnum"=w277) -> ()  [unwired: 2 in, 2 out]
            n103 = property on="HRME Exposure" class="Slide (strict)"("DisabledEnum"=w277) -> ()  [unwired: 2 in, 2 out]
            n104 = property on="Calibrate" class="Bool"("DisabledEnum"=w277) -> ()  [unwired: 2 in, 2 out]
            n105 = property on="HRME Gain" class="Slide (strict)"("DisabledEnum"=w277) -> ()  [unwired: 2 in, 2 out]
            n106 = property on="Close Program" class="Bool"("DisabledEnum"=w277) -> ()  [unwired: 2 in, 2 out]
            n107 = property on="Auto Gain" class="Bool (strict)"("DisabledEnum"=w277) -> ()  [unwired: 2 in, 2 out]
            n108 = property on="Save Button" class="Bool"("DisabledEnum"=w277) -> ()  [unwired: 2 in, 2 out]
            n109 = property on="Auto Exposure" class="Bool (strict)"("DisabledEnum"=w277) -> ()  [unwired: 2 in, 2 out]
            n110 = local read "Auto Exposure"() -> (w272:bool)
            n111 = local read "Auto Gain"() -> (w273:bool)
            n112 = local read "HRME Exposure"() -> (w274:dbl)
            n113 = local read "HRME Gain"() -> (w275:dbl)
            n114 = local read "Log File Out"() -> (w276:refnum<file>)
            n115 = call "Esophageal_Datalogger_PlayButton.vi"("Gain Value"=w275, "Auto Exposure Status"=w272, "error in (no error)"=w271, "Exposure Value"=w274, "Auto Gain Status"=w273, "Log File In"=w276) -> ("error out"=w270:errorcluster)  [unwired: 4 in, 1 out]
          }
          event "Auto Gain": Value Change {
            # "Disable if autogain is turned on"
            # "Select on/off"
            # "Turn auto gain on or off"
            n116 = event-data() -> ("NewVal"=w288:bool)  [unwired: 1 in, 2 out]
            n117 = Select(t=u32 1 ("ValueU32"), s=w288, f=u32 0 ("ValueU32")) -> (s? t:f=w291:u32)
            n118 = Select(t=T4."Disabled and Grayed Out" ("Disabled"), s=w288, f=T4."Enabled" ("Disabled")) -> (s? t:f=w287:T4)
            n119 = property class="IMAQdx"(reference=w297, error in=w295, "ActiveAttribute"="CameraAttributes::AnalogControl::GainAuto", "ValueU32"=w291) -> (reference out=w296:T8, error out=w286:errorcluster)
            n120 = property on="HRME Gain" class="Slide (strict)"(error in=w286, "DisabledEnum"=w287) -> (error out=w285:errorcluster)  [unwired: 1 in, 1 out]
          }
          event "Auto Exposure": Value Change {
            # "Disable if autogain is turned on"
            n121 = event-data() -> ("NewVal"=w301:bool)  [unwired: 1 in, 2 out]
            n122 = Select(t=u32 1 ("ValueU32"), s=w301, f=u32 0 ("ValueU32")) -> (s? t:f=w313:u32)
            n123 = Select(t=T4."Disabled and Grayed Out" ("Disabled"), s=w301, f=T4."Enabled" ("Disabled")) -> (s? t:f=w302:T4)
            n124 = property class="IMAQdx"(reference=w310, error in=w308, "ActiveAttribute"="CameraAttributes::AcquisitionControl::ExposureAuto", "ValueU32"=w313) -> (reference out=w309:T8, error out=w304:errorcluster)
            n125 = property on="HRME Exposure" class="Slide (strict)"(error in=w304, "DisabledEnum"=w302) -> (error out=w303:errorcluster)  [unwired: 1 in, 1 out]
          }
          event "Close Program": Value Change {
            n126 = event-data() -> ()  [unwired: 1 in, 3 out]
          }
          event "HRME Exposure": Value Change {
            # "Change fastHRME Exposure"
            n127 = event-data() -> ()  [unwired: 1 in, 6 out]
            n128 = property class="IMAQdx"(reference=w325, error in=w321, "ActiveAttribute"="CameraAttributes::AcquisitionControl::ExposureTime", "ValueU32"="HRME Exposure") -> (reference out=w324:T8, error out=w320:errorcluster)
          }
          event "HRME Gain": Value Change {
            # "Change fastHRME Gain"
            n129 = event-data() -> ()  [unwired: 1 in, 6 out]
            n130 = property class="IMAQdx"(reference=w334, error in=w331, "ActiveAttribute"="CameraAttributes::AnalogControl::Gain", "ValueU32"="HRME Gain") -> (reference out=w333:T8, error out=w332:errorcluster)
          }
          event "Save Button": Value Change {
            w373 = u32 1 items=["Frame", "Fill", "Highlight"] ("Drawing Mode (Frame)")
            w389 = T11 0 items=["Grayscale (U8)", "Grayscale (I16)", "Grayscale (SGL)", "Complex (CSG)", "RGB (U32)", "HSL (U32)", "RGB (U64)", "Grayscale (U16)"] ("Image Type")
            # "location of python file"
            # "creat json file path 2 save img score"
            # "Log Image Params"
            # "Overlay Colored Box"
            # "Cast to External Monitor"
            # "Update Number of Images Acquired"
            # "Generate Filename"
            # "Acquire Image"
            # "Get Exposure and Gain Values"
            # "Save Image to File"
            n131 = event-data() -> ()  [unwired: 1 in, 6 out]
            n132 = local read "Saved Imaged Number"() -> (w391:i32)
            n133 = property class="IMAQdx"(reference=w385, "ActiveAttribute"="CameraAttributes::AcquisitionControl::ExposureTime", "ActiveAttribute"="CameraAttributes::AnalogControl::Gain") -> (reference out=w395:T8, "ValueU32"=w394:u32, "ValueU32"=w393:u32)  [unwired: 1 in, 1 out]
            n134 = call "IMAQ Cast Image 2"("Image Src"=w384, "Image Type"=w389, "error in (no error)"=w383) -> ("Image Dst Out"=w388:T1, "error out"=w387:errorcluster)  [unwired: 11 in]
            n135 = local read "Representative Images"() -> (w358:path)
            n136 = Increment(x=w391) -> (x+1=w366:i32)
            n137 = call "Esophageal_Generate_Image_Filename.vi"("Image Number"=w366, "HRME Gain"=w393, "HRME Exposure"=w394) -> ("Notification Text"=→"Image Save Notification":string, "Image Filename"=w359:string)  [unwired: 7 in]
            n138 = Build Path(base path=w358, name or relative path=w359) -> (appended path=w400:path)
            n139 = property class="Enum (strict)"(reference=w367) -> ("Value"=w368:enum16{"15.9", "24.0"})  [unwired: 1 in, 2 out]
            n140 = local write "Saved Imaged Number"(w366) -> ()
            n141 = call-poly "IMAQ Write File 2"("error in (no error)"=w387, "Image Quality"=u32 1000, "File Path"=w400, "Image"=w388) -> ("error out"=w351:errorcluster, "Image Out (duplicate)"=w398:T1)  [unwired: 6 in]
            n142 = case shown="\"15.9\", Default" w368 {
              tunnel: [15.9 24.0] -> w343
              frame "15.9", Default {
              }
              frame "24.0" {
              }
            }
            n143 = Build Path(base path=w358, name or relative path=w359) -> (appended path=w360:path)
            n144 = Search/Split String(string=w359, search string/char (-)=".") -> (substring before match=w363:string)  [unwired: 1 in, 2 out]
            n145 = Path To String(path=w360) -> (string=w354:string)
            n146 = Concatenate Strings(w363, ".json") -> (w362:string)
            n147 = local read "HRME Scores"() -> (w357:path)
            n148 = property on="Image Analysis Meter" class="Slide (strict)"("DisabledEnum"=T4."Enabled" ("Disabled")) -> ()  [unwired: 2 in, 2 out]
            n149 = Build Path(base path=path "C:/Users/EsophaHRME_Dell2/Documents/GitHub/Esophageal_HRME_Software/EsophagealDeployment/Multi_Task_Network", name or relative path="score_rep_img.py") -> (appended path=w352:path)
            n150 = Build Path(base path=w357, name or relative path=w362) -> (appended path=w361:path)
            n151 = Path To String(path=w361) -> (string=w348:string)
            n152 = node(w353, w352, "process_single_image", w351, "", w354, w348) -> (w337:refnum<k35>, w338:errorcluster, w339:string)  [unwired: 2 in, 2 out]
            n153 = Fract/Exp String To Number(string=w339) -> (number=w344:dbl)  [unwired: 3 in, 1 out]
            n154 = Multiply(x=w344, y=100.0) -> (x*y=w341:dbl)
            "Image Analysis Meter" <- w341
            n155 = Greater?(x=w341, y=w343) -> (0:w347:bool)
            n156 = Select(t=u32 16718848, s=w347, f=u32 65289) -> (s? t:f=w340:u32)
            n157 = property on="Image Analysis Meter" class="Slide (strict)"(error in=w338, "Fill Color"=w340) -> (error out=w371:errorcluster)  [unwired: 1 in, 1 out]
            n158 = local read "Timestamp"() -> (w372:string)
            n159 = local read "Log File Out"() -> (w369:refnum<file>)
            n160 = local read "HRME Image"() -> (w379:T1)
            n161 = call "Esophageal_Datalogger_SaveButton.vi"("HRME Score"=w339, "error in (no error)"=w371, "Timestamp"=w372, "Image Name"=w359, "Log File In"=w369) -> ("error out"=w370:errorcluster)  [unwired: 5 in, 1 out]
            n162 = call "IMAQ Overlay Rectangle"("Color"=w340, "Group"=w339, "error in (no error)"=w370, "Drawing Mode (Frame)"=w373, "Rectangle"=T7 {"Left"=0, "Top"=0, "Right"=50, "Bottom"=50}, "Image"=w379) -> ("error out"=w375:errorcluster, "Image Out"=w378:T1)  [unwired: 4 in]
            n163 = local read "Height"() -> (w382:i16)
            n164 = call "IMAQ Merge Overlay"("error in (no error)"=w375, "Image Src"=w378) -> ("error out"=w376:errorcluster, "Image Dst Out"=w377:T1)  [unwired: 8 in]
            n165 = local read "Width"() -> (w381:i16)
            n166 = call "Esophageal_CastImage.vi"("X Resolution"=w381, "Y Resolution"=w382, "error in (no error)"=w376, "Image In"=w377) -> ("error out"=w380:errorcluster)  [unwired: 7 in]
          }
        }
        n167 = call-poly <vilib>:"DAQmx Read.vi"("task/channels in"=w158, "error in"=w142) -> ("task out"=w154:refnum<k21>, "data"=w157:bool[], "error out"=w149:errorcluster)  [unwired: 11 in]
        n168 = Index Array(array=w157, index=0) -> (element=w156:bool)
        n169 = Not(x=w156) -> (.not. x?=w155:bool)
        n170 = case shown="False" w155 {
          selector: w155 -> [w179 _]
          tunnel: w154 -> [w180 w194]
          tunnel: [w180 w193] -> w153
          tunnel: [w179 w192] -> w152
          tunnel: w149 -> [w178 w191]
          tunnel: [w178 w181] -> w148
          frame False {
          }
          frame True {
            w190 = T4."Disabled and Grayed Out" ("Disabled")
            # "Log Imaging Params"
            # "Enable the pause button"
            # "Disable all controls on the front panel except the pause button"
            # "Waits until the foot pedal is done being pressed."
            n171 = while {
              tunnel: w194 -> [w202]
              tunnel: [w201] -> w193
              tunnel: [w197] -> w192
              tunnel: w191 -> [w198]
              tunnel: [w195] -> w188
              stop <- w196 stop-if-true
              n172 = call-poly <vilib>:"DAQmx Read.vi"("task/channels in"=w202, "error in"=w198) -> ("task out"=w201:refnum<k21>, "data"=w199:bool[], "error out"=w195:errorcluster)  [unwired: 11 in]
              n173 = Index Array(array=w199, index=0) -> (element=w197:bool)
              n174 = Or(x=w197, y=w195) -> (x .or. y?=w196:bool)
            }
            n175 = property on="Play Button" class="Bool"("DisabledEnum"=w190) -> ()  [unwired: 2 in, 2 out]
            n176 = property on="Calibrate" class="Bool"("DisabledEnum"=w190) -> ()  [unwired: 2 in, 2 out]
            n177 = property on="Close Program" class="Bool"("DisabledEnum"=w190) -> ()  [unwired: 2 in, 2 out]
            n178 = property on="Save Button" class="Bool"("DisabledEnum"=w190) -> ()  [unwired: 2 in, 2 out]
            n179 = property on="HRME Exposure" class="Slide (strict)"("DisabledEnum"=w190) -> ()  [unwired: 2 in, 2 out]
            n180 = property on="HRME Gain" class="Slide (strict)"("DisabledEnum"=w190) -> ()  [unwired: 2 in, 2 out]
            n181 = property on="Pause Button" class="Bool"(error in=w188, "DisabledEnum"=T4."Enabled" ("Disabled")) -> (error out=w182:errorcluster)  [unwired: 1 in, 1 out]
            n182 = property on="Auto Gain" class="Bool (strict)"("DisabledEnum"=w190) -> ()  [unwired: 2 in, 2 out]
            n183 = property on="Auto Exposure" class="Bool (strict)"("DisabledEnum"=w190) -> ()  [unwired: 2 in, 2 out]
            n184 = local read "Auto Exposure"() -> (w183:bool)
            n185 = local read "Auto Gain"() -> (w184:bool)
            n186 = local read "HRME Exposure"() -> (w185:dbl)
            n187 = local read "HRME Gain"() -> (w186:dbl)
            n188 = local read "Log File Out"() -> (w187:refnum<file>)
            n189 = call "Esophageal_Datalogger_PlayButton.vi"("Gain Value"=w186, "Auto Exposure Status"=w183, "error in (no error)"=w182, "Exposure Value"=w185, "Auto Gain Status"=w184, "Log File In"=w187) -> ("error out"=w181:errorcluster)  [unwired: 4 in, 1 out]
          }
        }
        n190 = Select(t=Esophogeal_Software_States."Imaging" ("Anal HRME States"), s=w152, f=w161) -> (s? t:f=w162:T2)
        n191 = Merge Errors(w147, w148, w141) -> (w146:errorcluster)
      }
      frame "Imaging" {
        w413 = T11 4 items=["Grayscale (U8)", "Grayscale (I16)", "Grayscale (SGL)", "Complex (CSG)", "RGB (U32)", "HSL (U32)", "RGB (U64)", "Grayscale (U16)"] ("Image Type")
        # "Log Imaging Paused"
        # "Turn Red Light on to indicate frames are now being saved"
        n192 = while {
          tunnel: w430 -> [w520]
          tunnel: w429 -> [w519]
          tunnel: [w488] -> w428
          tunnel: [w498] -> w427
          tunnel: [w515] -> w411
          tunnel: w412 -> [w517]
          shift-right: [w512] -> w423
          shift-left: w426 -> [w518]
          tunnel: [w511] -> w422
          tunnel: [w509] -> w419
          tunnel: [w489] -> w414
          tunnel: [w487] -> w408
          stop <- w510 stop-if-true
          w495 = T4."Disabled and Grayed Out" ("Disabled")
          w496 = T11 0 items=["Grayscale (U8)", "Grayscale (I16)", "Grayscale (SGL)", "Complex (CSG)", "RGB (U32)", "HSL (U32)", "RGB (U64)", "Grayscale (U16)"] ("Image Type")
          # "Converts image to array"
          # "Generate filename from timestamp"
          # "Send to producer"
          # "Read Foot Pedal Status"
          # "Acquire fastHRME Image"
          n193 = call <vilib>:"IMAQdx Grab2.vi"("error in"=w517, "Image In"=w519, "Session In"=w520) -> ("error out"=w497:errorcluster, "Image Out"=w498:T1, "Session Out"=w488:T8)  [unwired: 5 in, 1 out]
          n194 = call "IMAQ Cast Image 2"("Image Src"=w498, "Image Type"=w496, "error in (no error)"=w497) -> ("Image Dst Out"=w492:T1, "error out"=w491:errorcluster)  [unwired: 11 in]
          n195 = local read "Height"() -> (w494:i16)
          n196 = local write "HRME Image"(w492) -> ()
          n197 = Format Date/Time String(time format string (%c)="%H%M%S%3u") -> (date/time string=w501:string)  [unwired: 2 in]
          n198 = local read "Width"() -> (w493:i16)
          n199 = call "IMAQ ImageToArray"("Image"=w492) -> ("Image Pixels (U8)"=w502:u8[][])  [unwired: 3 in, 4 out]
          n200 = call-poly <vilib>:"DAQmx Read.vi"("task/channels in"=w518, "error in"=w517) -> ("task out"=w504:refnum<k21>, "data"=w506:bool[], "error out"=w503:errorcluster)  [unwired: 11 in]
          n201 = call "Esophageal_CastImage.vi"("X Resolution"=w493, "Y Resolution"=w494, "error in (no error)"=w491, "Image In"=w492) -> ("error out"=w490:errorcluster)  [unwired: 7 in]
          n202 = Concatenate Strings(w501, ".png" ("string")) -> (w487:string)
          n203 = call <extravilib>:"Write.vi"("element"=w487) -> ("channel"=w509:T13)  [unwired: 8 in, 2 out]
          n204 = Index Array(array=w506, index=0) -> (element=w507:bool)
          n205 = Not(x=w507) -> (.not. x?=w505:bool)
          n206 = case shown="True" w505 {
            selector: w505 -> [w522 _]
            tunnel: w504 -> [w523 w528]
            tunnel: [w523 w527] -> w512
            tunnel: [w522 w524] -> w513
            tunnel: w503 -> [w521 w526]
            tunnel: [w521 w525] -> w516
            frame False {
            }
            frame True {
              # "Waits until the foot pedal is done being pressed."
              n207 = while {
                tunnel: w528 -> [w535]
                tunnel: [w534] -> w527
                tunnel: [w531] -> w524
                tunnel: w526 -> [w530]
                tunnel: [w529] -> w525
                stop <- w531 stop-if-true
                n208 = call-poly <vilib>:"DAQmx Read.vi"("task/channels in"=w535, "error in"=w530) -> ("task out"=w534:refnum<k21>, "data"=w532:bool[], "error out"=w529:errorcluster)  [unwired: 11 in]
                n209 = Index Array(array=w532, index=0) -> (element=w531:bool)
              }
            }
          }
          n210 = property on="Save Button" class="Bool"("DisabledEnum"=w495) -> ()  [unwired: 2 in, 2 out]
          n211 = property on="Play Button" class="Bool"("DisabledEnum"=w495) -> ()  [unwired: 2 in, 2 out]
          n212 = property on="Image Analysis Meter" class="Slide (strict)"("DisabledEnum"=w495) -> ()  [unwired: 2 in, 2 out]
          n213 = Or(x="Pause Button", y=w513) -> (x .or. y?=w510:bool)
          "Pause Status" <- w510
          n214 = call <extravilib>:"Write.vi"("last element? (F)"=w510, "element"=w502) -> ("channel"=w511:T14)  [unwired: 7 in, 2 out]
          n215 = Merge Errors(w490, w516) -> (w515:errorcluster)
          n216 = call <extravilib>:"Write.vi"("element"=w510) -> ("channel"=w489:T15)  [unwired: 1 out]
        }
        "Timestamp" <- w408
        n217 = while {
          shift-right: [w463] -> _
          shift-left: w406 -> [w462]
          shift-right: [w456] -> _
          shift-left: w405 -> [w461]
          shift-right: [w453] -> w404
          shift-left: w407 -> [w460]
          tunnel: [w459] -> w417
          tunnel: [w458] -> w416
          tunnel: w414 -> [w457]
          i -> [w449]
          stop <- w446 stop-if-true
          # "Attempt to slow down frame rate"
          n218 = call <vilib>:"IMAQdx Grab2.vi"("error in"=w460, "Image In"=w461, "Session In"=w462) -> ("error out"=w455:errorcluster, "Image Out"=w456:T1, "Session Out"=w463:T8)  [unwired: 5 in, 1 out]
          n219 = call <extravilib>:"Read.vi"("channel"=w457) -> ("element"=w446:bool)  [unwired: 1 in, 1 out]
          n220 = Quotient & Remainder(x=w449, y=4) -> (x-y*floor(x/y)=w447:i32)  [unwired: 1 out]
          n221 = Equal To 0?(x=w447) -> (x = 0?=w445:bool)
          n222 = Or(x=w445, y=w446) -> (x .or. y?=w444:bool)
          n223 = call "IMAQ Resample"("X Resolution"=960, "Y Resolution"=540, "error in (no error)"=w455, "Image Src"=w456) -> ("error out"=w454:errorcluster, "Image Dst Out"=w452:T1)  [unwired: 6 in]
          "Endoscope Feed" <- w452
          n224 = case shown="True" w444 {
            tunnel: [_ w474] -> w459
            tunnel: [_ w469] -> w458
            tunnel: w446 -> [_ w465]
            tunnel: w454 -> [w464 w468]
            tunnel: [w464 w467] -> w453
            tunnel: w452 -> [_ w466]
            frame False {
            }
            frame True {
              n225 = Format Date/Time String(time format string (%c)="%H%M%S%3u") -> (date/time string=w471:string)  [unwired: 2 in]
              n226 = call "IMAQ ColorImageToArray"("Image"=w466, "error in (no error)"=w468) -> ("Image Pixels (U32)"=w475:u32[][], "error out"=w467:errorcluster)  [unwired: 2 in, 1 out]
              n227 = Concatenate Strings(w471, ".png" ("string")) -> (w470:string)
              n228 = call <extravilib>:"Write.vi"("last element? (F)"=w465, "element"=w475) -> ("channel"=w474:T16)  [unwired: 7 in, 2 out]
              n229 = call <extravilib>:"Write.vi"("last element? (F)"=w465, "element"=w470) -> ("channel"=w469:T13)  [unwired: 7 in, 2 out]
            }
          }
        }
        n230 = call "IMAQ Create"("Image Name"="Endoscope Consumer", "Image Type"=w413) -> ("New Image"=w415:T1)  [unwired: 3 in, 1 out]
        n231 = call "IMAQ Create"("Image Name"="HRME Consumer") -> ("New Image"=w420:T1)  [unwired: 4 in, 1 out]
        n232 = while {
          tunnel: w417 -> [w443]
          tunnel: w416 -> [w442]
          shift-right: [w435] -> _
          shift-left: w415 -> [w440]
          stop <- w433 stop-if-true
          # "Take filename from channel"
          # "Take image from channel"
          # "Save the image to file"
          # "Reads image from channel, converts it into an image, then writes that image to file."
          n233 = local read "WideField Path"() -> (w439:path)
          n234 = call <extravilib>:"Read.vi"("channel"=w443) -> ("done?"=w433:bool, "element"=w441:u32[][])  [unwired: 6 in, 3 out]
          n235 = call <extravilib>:"Read.vi"("channel"=w442) -> ("element"=w438:string)  [unwired: 6 in, 4 out]
          n236 = call "IMAQ ArrayToColorImage"("Image Pixels (U32)"=w441, "Image"=w440) -> ("Image Out"=w436:T1)  [unwired: 3 in, 1 out]
          n237 = Build Path(base path=w439, name or relative path=w438) -> (appended path=w434:path)
          n238 = call-poly "IMAQ Write File 2"("Image Quality"=u32 1000, "File Path"=w434, "Image"=w436) -> ("Image Out (duplicate)"=w435:T1)  [unwired: 7 in, 1 out]
        }
        n239 = while {
          tunnel: w422 -> [w486]
          shift-right: [w482] -> _
          shift-left: w420 -> [w478]
          tunnel: w419 -> [w481]
          stop <- w485 stop-if-true
          # "Reads image from channel, converts it into an image, then writes that image to file."
          n240 = local read "HRME Path"() -> (w477:path)
          n241 = call <extravilib>:"Read.vi"("channel"=w486) -> ("done?"=w485:bool, "element"=w484:u8[][])  [unwired: 6 in, 3 out]
          n242 = call <extravilib>:"Read.vi"("channel"=w481) -> ("element"=w479:string)  [unwired: 6 in, 4 out]
          n243 = call "IMAQ ArrayToImage"("Image Pixels (U8)"=w484, "Image"=w478) -> ("Image Out"=w483:T1)  [unwired: 8 in, 1 out]
          n244 = Build Path(base path=w477, name or relative path=w479) -> (appended path=w480:path)
          n245 = call-poly "IMAQ Write File 2"("Image Quality"=u32 1000, "File Path"=w480, "Image"=w483) -> ("Image Out (duplicate)"=w482:T1)  [unwired: 7 in, 1 out]
        }
        n246 = local read "Log File Out"() -> (w409:refnum<file>)
        n247 = call "Esophageal_Datalogger_PauseButton.vi"("error in (no error)"=w411, "Log File In"=w409) -> ("error out"=w410:errorcluster)  [unwired: 8 in, 1 out]
        "Recording" <- TRUE ("Recording")
      }
      frame "Exit" {
        # "Log Program Finished"
        # "Tell the python program to close"
        n248 = Bundle By Name(cluster=T6 {"Source"="", "Destination"="", "CMD"="newfolders", "Time"="time"} ("Output JSON File"), "CMD"="stop") -> (w548:T6)
        n249 = local read "Command File Location"() -> (w545:path)
        n250 = Flatten To JSON(anything=w548, error in (no error)=w543) -> (JSON string=w547:string, 11:w546:errorcluster)  [unwired: 1 in]
        n251 = Write to Text File(file (use dialog)=w545, text=w547, error in=w546) -> (error out=w542:errorcluster)  [unwired: 1 in, 2 out]
        n252 = local read "Log File Out"() -> (w540:refnum<file>)
        n253 = call "Esophageal_Datalogger_EndButton.vi"("error in (no error)"=w542, "Log File In"=w540) -> ("error out"=w541:errorcluster)  [unwired: 8 in, 1 out]
      }
    }
    "Software States" <- w33
    "error out" <- w25
  }
  n254 = property on="Play Button" class="Bool"("DisabledEnum"=w3) -> ()  [unwired: 2 in, 2 out]
  n255 = property on="Calibrate" class="Bool"("DisabledEnum"=w3) -> ()  [unwired: 2 in, 2 out]
  n256 = property on="Save Button" class="Bool"("DisabledEnum"=w3) -> ()  [unwired: 2 in, 2 out]
  n257 = property on="Close Program" class="Bool"("DisabledEnum"=w3) -> ()  [unwired: 2 in, 2 out]
  n258 = property on="Auto Exposure" class="Bool (strict)"("DisabledEnum"=w3) -> ()  [unwired: 2 in, 2 out]
  n259 = property on="Auto Gain" class="Bool (strict)"("DisabledEnum"=w3) -> ()  [unwired: 2 in, 2 out]
  n260 = property on="Image Analysis Meter" class="Slide (strict)"("BG Color"=u32 0 ("Slider Colors:BG Color")) -> ()  [unwired: 2 in, 2 out]
  n261 = call <vilib>:"DAQmx Clear Task.vi"("task in"=w10, "error in"=w9) -> ("error out"=w1:errorcluster)  [unwired: 13 in]
  n262 = Close Python Session(session in=w2, error in=w1) -> ()  [unwired: 1 out]
